vi "Steuerprogramm-11-15.vi"() -> ()   [LabVIEW 2010]
uses:
  <vilib>/rvi/interface/nirviReadWriteControl/nirviReadWriteControl.xnode
  <vilib>/rvi/errors/niLvFpgaWhatHappensToTopLevelVI.ctl
  <vilib>/rvi/interface/common/niFpgaNodeNameForErrorReporting.ctl
  <vilib>/rvi/errors/niLvFpgaAdjustHostInterfaceError.vi
  gvbooleschRT.vi
  <vilib>/functionblocks/FB Core/FB Core.xnode
  <vilib>/functionblocks/Counter/Elapsed Timer/Elapsed Timer.vi
  <vilib>/functionblocks/NI_FunctionBlock Libraries.lvlib
  <vilib>/rvi/interface/nirviCloseFPGA/nirviCloseFPGA.xnode
  <vilib>/addons/control/pid/NI_PID_pid.lvlib
  GVMWHorst.vi
  GVMethodenwechsel.vi
  GVHorstSP.vi
  GVZwangs.vi
  GVHK1Hz.vi
  GVHeizenLH.vi
  GVAIs.vi
  <vilib>/addons/control/pid/pid.llb/PID (DBL Array).vi
  GVTrapsMachs.vi
  GVaktuelleTDMS.vi
  GVECDs.vi
  GVZeitenZyklen.vi
  GVProbenvol.vi
  GVVentilposition.vi
  <vilib>/rvi/interface/nirviMethod/nirviMethod.xnode
  GVChroms.vi
  C:/Users/HAGAR-IV/Desktop/Zeugs/Johnny/pertrasgc fpga/FPGA-Programm-11-15.vi
  NiFpgaLv.dll
  <vilib>/Utility/error.llb/Error Cluster From Error Code.vi
  C:/Users/HAGAR-IV/Desktop/Zeugs/markus/version feb 2012/FPGA Bitfiles/pertrasgcfpga2_FPGATarget_FPGA-Programm-11_875D3646.lvbitx
  <vilib>/FPGAPlugInAG/cRIO-9114/niLvFpga_Close_cRIO-9114.vi
  Emil/HAGAR V - Licor/control/Licor-Sequences.ctl
  Emil/HAGAR V - Licor/control/Licor-Pump.ctl
  Emil/Licor-Steuerung/LicorLI7000/conventions/Licor-Source.ctl
  Emil/Licor-Steuerung/LicorLI7000/LicorLI7000.lvlib
panel:
  in  "Methode speichern":bool
  out "ZyklusNummernGesamt":i32[](array[numeric])
  in  "veränderte Methode benutzen":bool
  in  "Methode verändern":bool
  out "ZyklusNummern":i32[](array[numeric])
  out "Big Ben, Methodenzeit, Zykluszeit0, Zykluszeit1, Zykluszeit2A, Zykluszeit2B":i32[](array[numeric])
  in  "global stop RT":bool
  in  "Methode":i32(ring) items=["Bedingsmethode", "Startmethode", "Meßmodus", "Shut-up-Methode", "Test"]
  in  "Registerkarte":T1(tab)
  out "AIs1":dbl[](array[numeric])
  out "AIs1":string[](array[string])
  out "AIs2":string[](array[string])
  out "AIs3":string[](array[string])
  out "AIs2":dbl[](array[numeric])
  out "AIs3":dbl[](array[numeric])
  out "schnelleAnzeige":cluster{dbl[], dbl[]}(graph)
  in  "TafelWischen!":bool
  in  "dargestellte Größe 3":i32(ring)=1 items=["TemperaturTrap1[°C]", "TemperaturTrap2[°C]", "TemperaturPreMach1[°C]", "TemperaturPreMach2[°C]", "TemperaturMainMach1[°C]", "TemperaturMainMach2[°C]", "PrC0", "PrC0-Licor", "PrC1-Säule2", "PrC1-Säule1", "MFC1-Sample", "MFC1-Methan", "PrC1-BackFlush1", "PrC1-BackFlush2", "MFC2A", "MFC2B", "MFC2C", "PrC2A", "MFC2D", "MFC2E", "PrC2B"]
  in  "An/Aus":bool
  out "CO2 B 2":cluster{"t0":dbl, "dt":dbl, "Y":dbl[]}(graph)
  in  "manual control":T3={"sequence manual"=enum."WAIT", "sequence manual ?"=FALSE}
  out "raw data buffer out":string[](array[string])
  in  "command parameter":T6={"CO2 ref"=392.0, "CO2 span"=372.0, "H2O ref"=0.0, "H2O span"=0.0, "Zt"=0.0, "Zi"=1.2, "Zeitstempel"=timestamp(0 s since 1904-01-01), "Zm"=0.0, "Licor-Pump"="Off", "Licor-Sources"=["CO2A W", "CO2B W", "H2OA W", "H2OB W", "T C", "T V", "P kPa", "P V", "RH %", "CO2A um/m", "CO2B um/m", "H2OA mm/m", "H2OB mm/m"], "S"=1.0}
  out "Housekeeping1":cluster{dbl[], dbl[]}(graph)
  in  "Zeitachse1":i32(ring)=1 items=["Zykluszeit [s] Mod0", "Zykluszeit [s] Mod1", "Zykluszeit [s] Mod2A", "Zykluszeit [s] Mod2B"]
  in  "dargestellte Größe 1":i32(ring)=1 items=["T1-Trap1", "T1-Trap2", "T1-StirlingKühlkopf", "T1-PreCol1", "T1-PreCol2", "T1-MainCol1a", "T1-MainCol1b", "T1-MainCol2a", "T1-MainCol2b", "T1-Bronkhorst1a", "T1-Bronkhorst1b", "T1-Bronkhorst2a", "T1-Bronkhorst2b", "T1-2Pos1B", "T1-Spare9", "T1-2Pos1A", "T1-Spare10", "T1-TurboPump", "T1-StirlingPlatine", "T1-Spare5", "T1-Spare6", "T1-Spare7", "T1-Spare8", "F1-MFM1", "F1-MFM0D [mL]", "P1-MethaneHP", "P1-MethaneLP", "P1-Vacuum", "TurboSpeed", "I1-MS-AC", "I1-Trap1", "I1-Trap2", "T2-ECD1a", "T2-ECD1b", "T2-ECD2a", "T2-ECD2b", "T2-Col1a", "T2-Col1b", "T2-Col2a", "T2-Col2b", "T2-Spare1", "T2-Spare2", "T2-Oven_a", "T2-Oven_b", "T2-Spare3", "T2-Spare4", "T2-Spare5", "F2-MFM0", "F2-MFM2A", "F2-MFM2B", "P2-N2O_HP", "P2-N2O_LP", "P2-CO2_HP", "P2-CO2_LP", "AI-Spare1", "FL-MFM1000mL", "AI-Spare3", "AI-Spare4", "AI-Spare5", "AI-Spare6", "AI-Spare7", "AI-Spare8", "AI-Spare9", "FL-MFM30mL", "T0-DC/DC5", "I0-24V_M0", "I0-48V_M1", "I0-24V_M1", "I0-28V_M2", "T0-Spare3", "T0-Spare2", "T0-Spare4", "T0-DC/DC7", "I0-20V_Laptop", "I0-28V_M1", "I0-24V_M2", "I0-12V_Licor", "T0-Spare1", "T0-Drier", "T0-Spare5", "F0-MFM0A [L]", "TL-Licor_a", "P0-Span-HP", "P0-spare1", "P0-Stickstoff-LP", "P0-Helium-LP", "P0-Cal-HP", "P0-P9Tavco[bar]", "F0-MFM0B [L]", "TL-Licor_b", "P0-Span-LP", "P0-spare2", "P0-Stickstoff-HP", "P0-Helium-HP", "P0-Cal-LP", "F0-MFM3", "TemperaturTrap1[°C]", "TemperaturTrap2[°C]", "TemperaturPreMach1[°C]", "TemperaturPreMach2[°C]", "TemperaturMainMach1[°C]", "TemperaturMainMach2[°C]", "PrC0", "PrC0-Licor", "PrC1-Säule2", "PrC1-Säule1", "MFC1-Sample", "MFC1-Methan", "PrC1-BackFlush1", "PrC1-BackFlush2", "MFC2A", "MFC2B", "MFC2C", "PrC2A", "MFC2D", "MFC2E", "PrC2B"]
  out "Housekeeping2":cluster{dbl[], dbl[]}(graph)
  in  "Zeitachse2":i32(ring)=1 items=["Zykluszeit [s] Mod0", "Zykluszeit [s] Mod1", "Zykluszeit [s] Mod2A", "Zykluszeit [s] Mod2B"]
  in  "dargestellte Größe 2":i32(ring)=1 items=["T1-Trap1", "T1-Trap2", "T1-StirlingKühlkopf", "T1-PreCol1", "T1-PreCol2", "T1-MainCol1a", "T1-MainCol1b", "T1-MainCol2a", "T1-MainCol2b", "T1-Bronkhorst1a", "T1-Bronkhorst1b", "T1-Bronkhorst2a", "T1-Bronkhorst2b", "T1-2Pos1B", "T1-Spare9", "T1-2Pos1A", "T1-Spare10", "T1-TurboPump", "T1-StirlingPlatine", "T1-Spare5", "T1-Spare6", "T1-Spare7", "T1-Spare8", "F1-MFM1", "F1-MFM0D [mL]", "P1-MethaneHP", "P1-MethaneLP", "P1-Vacuum", "TurboSpeed", "I1-MS-AC", "I1-Trap1", "I1-Trap2", "T2-ECD1a", "T2-ECD1b", "T2-ECD2a", "T2-ECD2b", "T2-Col1a", "T2-Col1b", "T2-Col2a", "T2-Col2b", "T2-Spare1", "T2-Spare2", "T2-Oven_a", "T2-Oven_b", "T2-Spare3", "T2-Spare4", "T2-Spare5", "F2-MFM0", "F2-MFM2A", "F2-MFM2B", "P2-N2O_HP", "P2-N2O_LP", "P2-CO2_HP", "P2-CO2_LP", "AI-Spare1", "FL-MFM1000mL", "AI-Spare3", "AI-Spare4", "AI-Spare5", "AI-Spare6", "AI-Spare7", "AI-Spare8", "AI-Spare9", "FL-MFM30mL", "T0-DC/DC5", "I0-24V_M0", "I0-48V_M1", "I0-24V_M1", "I0-28V_M2", "T0-Spare3", "T0-Spare2", "T0-Spare4", "T0-DC/DC7", "I0-20V_Laptop", "I0-28V_M1", "I0-24V_M2", "I0-12V_Licor", "T0-Spare1", "T0-Drier", "T0-Spare5", "F0-MFM0A [L]", "TL-Licor_a", "P0-Span-HP", "P0-spare1", "P0-Stickstoff-LP", "P0-Helium-LP", "P0-Cal-HP", "P0-P9Tavco[bar]", "F0-MFM0B [L]", "TL-Licor_b", "P0-Span-LP", "P0-spare2", "P0-Stickstoff-HP", "P0-Helium-HP", "P0-Cal-LP", "F0-MFM3", "TemperaturTrap1[°C]", "TemperaturTrap2[°C]", "TemperaturPreMach1[°C]", "TemperaturPreMach2[°C]", "TemperaturMainMach1[°C]", "TemperaturMainMach2[°C]", "PrC0", "PrC0-Licor", "PrC1-Säule2", "PrC1-Säule1", "MFC1-Sample", "MFC1-Methan", "PrC1-BackFlush1", "PrC1-BackFlush2", "MFC2A", "MFC2B", "MFC2C", "PrC2A", "MFC2D", "MFC2E", "PrC2B"]
  out "Detektor 2":cluster{dbl[], dbl[]}[](graph)
  in  "Detektor":i32(ring) items=["ECD1", "ECD2"]
  in  "HK1YMin":dbl
  in  "HK1YMax":dbl=100.0
  in  "HK2YMin":dbl
  in  "HK2YMax":dbl=100.0
  in  "DetYMin":dbl
  in  "DetYMax":dbl=100.0
  out "Zykluslängen [s]":dbl[](array[numeric])
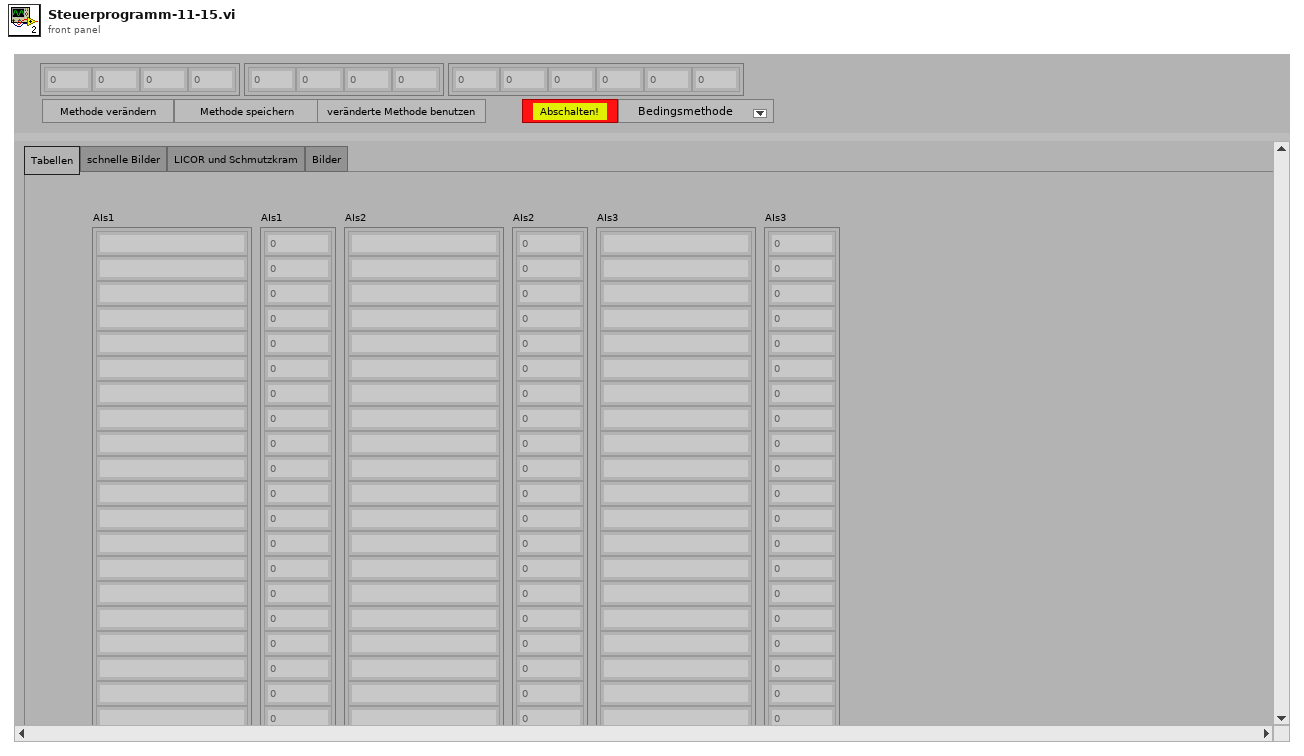
[diagram p1: front panel]
types:
  T1 = enum32{"Tabellen", "schnelle Bilder", "LICOR und Schmutzkram", "Bilder"}
  T2 = typedef "Licor-Sequences.ctl" = enum16{"test", "WAIT", "warmup", "initialize", "calibrate Z", "calibrate S"}
  T3 = cluster{"sequence manual":T2, "sequence manual ?":bool}
  T4 = typedef "Licor-Pump.ctl" = string
  T5 = typedef "LicorLI7000.lvlib/Licor-Source.ctl" = string
  T6 = cluster{"CO2 ref":dbl, "CO2 span":dbl, "H2O ref":dbl, "H2O span":dbl, "Zt":dbl, "Zi":dbl, "Zeitstempel":timestamp, "Zm":dbl, "Licor-Pump":T4, "Licor-Sources":T5[], "S":dbl}
  T7 = cluster{"Zykluslängen [s]":dbl[], "ZeitpktDIOsMod0":dbl[], "ZeitpktDIOsMod1":dbl[], "ZeitpktDIOsMod2A":dbl[], "ZeitpktDIOsMod2B":dbl[], "DIOsSPMod0":bool[][], "DIOsSPMod1":bool[][], "DIOsSPMod2A":bool[][], "DIOsSPMod2B":bool[][], "Mod0HorstZeitpkt":dbl[], "Mod1HorstZeitpkt":dbl[], "Mod2AHorstZeitpkt":dbl[], "Mod2BHorstZeitpkt":dbl[], "HorstSPMod0":dbl[][], "HorstSPMod1":dbl[][], "HorstSPMod2A":dbl[][], "HorstSPMod2B":dbl[][], "LHSetpoints":dbl[], "LHHeizen?":bool[], "ZPktFPGABoolesch":dbl[], "FPGABoolesch":bool[][], "ZeitpktFPGAPID":dbl[], "FPGAPID":cluster{"proportional gain (Kc)":fxp<+/-,16,8>, "integral gain (Kc*Ts/Ti)":fxp<+/-,16,8>, "derivative gain (Kc*Td/Ts)":fxp<+/-,16,8>}[][], "ZeitpktFPGAFixp":dbl[], "SHSetpoints":dbl[][], "t_PreMach1":dbl[], "T_PreMach1":dbl[], "t_PreMach2":dbl[], "T_PreMach2":dbl[], "PIDs für \"träge\" Heizungen":cluster{"proportional gain (Kc)":dbl, "integral time (Ti, min)":dbl, "derivative time (Td, min)":dbl}[], "Zwangsbedingungen":dbl[][], "Dateien fürs MS schicken?":bool, "ZeitpunkteMPV":dbl[], "SPMPV":i32[], "ZeitpktMS-1":dbl, "ZeitpktMS-2":dbl, "Int.Start1":dbl, "Int.Stop1":dbl, "Int.Start2":dbl, "Int.Stop2":dbl, "Methodenname":string, "t_MainMach1":dbl[], "T_MainMach1":dbl[], "t_MainMach2":dbl[], "T_MainMach2":dbl[]}[]
  T8 = cluster{"DIOsMod0Nr":i32[], "DIOsMod1Nr":i32[], "DIOsMod2ANr":i32[], "DIOsMod2BNr":i32[], "AIsLH":i32[], "Anzahl Horst/Modul":i32[], "Regler für den Probenfluß":i32, "StringSPvorgebenMod0":string[], "StringSPvorgebenMod1":string[], "StringSPvorgebenMod2A":string[], "StringSPvorgebenMod2B":string[], "StringMWAntwort0":string[], "StringMWAntwort1":string[], "StringMWAntwort2A":string[], "StringMWAntwort2B":string[], "UmrechnungHorst0":dbl[], "UmrechnungHorst1":dbl[], "UmrechnungHorst2A":dbl[], "UmrechnungHorst2B":dbl[], "StringMWabfragenMod0":string[], "StringMWabfragenMod1":string[], "StringMWabfragenMod2A":string[], "StringMWabfragenMod2B":string[], "Modul1/AI koeff":dbl[][], "Modul2/AI koeff":dbl[][], "Modul3/AI koeff":dbl[][], "Traps/MachsKoeff":dbl[][], "Modul1/AIsNamen":string[], "Modul2/AIsNamen":string[], "Modul3/AIsNamen":string[], "DIOsMod0Name":string[], "DIOsMod1Name":string[], "DIOsMod2AName":string[], "DIOsMod2BName":string[], "HorstMod0Name":string[], "HorstMod1Name":string[], "HorstMod2AName":string[], "HorstMod2BName":string[], "Startmethode":i32, "Dateiordner Housekeeping":path, "Dateiname Housekeeping":string, "DateiordnerECD1":path, "DateinameECD1":string, "DateiordnerECD2":path, "DateinameECD2":string, "NamenLangsameHeizungen":string[], "ModuleLH":i32[]}
  T9 = enum16{"open", "replace", "create", "open or create", "replace or create", "replace or create with confirmation"}
  T10 = cluster{"Zykluslängen [s]":dbl[], "ZeitpktDIOsMod0":dbl[], "ZeitpktDIOsMod1":dbl[], "ZeitpktDIOsMod2A":dbl[], "ZeitpktDIOsMod2B":dbl[], "DIOsSPMod0":bool[][], "DIOsSPMod1":bool[][], "DIOsSPMod2A":bool[][], "DIOsSPMod2B":bool[][], "Mod0HorstZeitpkt":dbl[], "Mod1HorstZeitpkt":dbl[], "Mod2AHorstZeitpkt":dbl[], "Mod2BHorstZeitpkt":dbl[], "HorstSPMod0":dbl[][], "HorstSPMod1":dbl[][], "HorstSPMod2A":dbl[][], "HorstSPMod2B":dbl[][], "LangsameHeizungenSP":dbl[], "LHHeizen?":bool[], "ZPktFPGABoolesch":dbl[], "FPGABoolesch":bool[][], "ZeitpktFPGAPID":dbl[], "FPGAPID":cluster{"proportional gain (Kc)":fxp<+/-,16,8>, "integral gain (Kc*Ts/Ti)":fxp<+/-,16,8>, "derivative gain (Kc*Td/Ts)":fxp<+/-,16,8>}[][], "ZeitpktFPGAFixp":dbl[], "FPGAFixp":fxp<+/-,16,4>[][], "ZeitpktMach1":dbl[], "TempMach1":dbl[], "ZeitpktMach2":dbl[], "TempMach2":dbl[], "PIDs für \"träge\" Heizungen":cluster{"proportional gain (Kc)":dbl, "integral time (Ti, min)":dbl, "derivative time (Td, min)":dbl}[], "Zwangsbedingungen":dbl[][], "Text0 MS-Datei":string, "Info":string, "wie wird gespeichert?":u16, "Speicherlänge":string, "Dateien fürs MS schicken?":bool, "Pfad MS-Datei CRIO":path}[]
  T11 = typedef "niFpgaNodeNameForErrorReporting.ctl" = enum16{"Open FPGA VI Reference", "Read/Write Control", "Invoke Method: Abort", "Invoke Method: Acknowledge IRQ", "Invoke Method: Download", "Invoke Method: FIFO.Configure", "Invoke Method: FIFO.Read", "Invoke Method: FIFO.Start", "Invoke Method: FIFO.Stop", "Invoke Method: FIFO.Write", "Invoke Method: Reset", "Invoke Method: Run", "Invoke Method: Wait on IRQ", "Close FPGA VI Reference"}
  T12 = typedef "niLvFpgaWhatHappensToTopLevelVI.ctl" = enum16{"top level VI scripted behind XNode", "top level VI inlined behind XNode"}
  T13 = cluster{"Zyklus1":i32, "Zeitachse1":i32, "dargestellte Größe 1":i32, "Zyklus2":i32, "Zeitachse2":i32, "dargestellte Größe 2":i32}
  T14 = cluster{"Zykluslängen [s]":dbl[], "ZeitpktDIOsMod0":dbl[], "ZeitpktDIOsMod1":dbl[], "ZeitpktDIOsMod2A":dbl[], "ZeitpktDIOsMod2B":dbl[], "DIOsSPMod0":bool[][], "DIOsSPMod1":bool[][], "DIOsSPMod2A":bool[][], "DIOsSPMod2B":bool[][], "Mod0HorstZeitpkt":dbl[], "Mod1HorstZeitpkt":dbl[], "Mod2AHorstZeitpkt":dbl[], "Mod2BHorstZeitpkt":dbl[], "HorstSPMod0":dbl[][], "HorstSPMod1":dbl[][], "HorstSPMod2A":dbl[][], "HorstSPMod2B":dbl[][], "LHSetpoints":dbl[], "LHHeizen?":bool[], "ZPktFPGABoolesch":dbl[], "FPGABoolesch":bool[][], "ZeitpktFPGAPID":dbl[], "FPGAPID":cluster{"proportional gain (Kc)":fxp<+/-,16,8>, "integral gain (Kc*Ts/Ti)":fxp<+/-,16,8>, "derivative gain (Kc*Td/Ts)":fxp<+/-,16,8>}[][], "ZeitpktFPGAFixp":dbl[], "SHSetpoints":dbl[][], "t_PreMach1":dbl[], "T_PreMach1":dbl[], "t_PreMach2":dbl[], "T_PreMach2":dbl[], "PIDs für \"träge\" Heizungen":cluster{"proportional gain (Kc)":dbl, "integral time (Ti, min)":dbl, "derivative time (Td, min)":dbl}[], "Zwangsbedingungen":dbl[][], "Dateien fürs MS schicken?":bool, "ZeitpunkteMPV":dbl[], "SPMPV":i32[], "ZeitpktMS-1":dbl, "ZeitpktMS-2":dbl, "Int.Start1":dbl, "Int.Stop1":dbl, "Int.Start2":dbl, "Int.Stop2":dbl, "Methodenname":string, "t_MainMach1":dbl[], "T_MainMach1":dbl[], "t_MainMach2":dbl[], "T_MainMach2":dbl[]}
  T15 = cluster{"DIOsMod0Name":string[], "DIOsMod1Name":string[], "DIOsMod2AName":string[], "DIOsMod2BName":string[], "HorstMod0Name":string[], "HorstMod1Name":string[], "HorstMod2AName":string[], "HorstMod2BName":string[], "NamenLangsameHeizungen":string[]}
  T16 = cluster{"Dateiordner Housekeeping":path, "DateiordnerECD1":path, "DateiordnerECD2":path, "Dateiname Housekeeping":string, "DateinameECD1":string, "DateinameECD2":string, "tdms0":refnum<k34>, "tdms1":refnum<k34>, "tdms0":refnum<k34>, "tdms1":refnum<k34>, "tdms0":refnum<k34>, "tdms1":refnum<k34>}
  T17 = cluster{"proportional gain (Kc)":fxp<+/-,16,8>, "integral gain (Kc*Ts/Ti)":fxp<+/-,16,8>, "derivative gain (Kc*Td/Ts)":fxp<+/-,16,8>}[][]
  T18 = cluster{"proportional gain (Kc)":dbl, "integral time (Ti, min)":dbl, "derivative time (Td, min)":dbl}[]
  T19 = cluster{"Heizen?LH[0]":bool, "Heizen?LH[1]":bool, "Heizen?LH[2]":bool, "Heizen?LH[3]":bool, "Heizen?LH[4]":bool, "Heizen?LH[5]":bool, "Heizen?LH[6]":bool, "Heizen?LH[7]":bool, "Heizen?LH[8]":bool, "Heizen?LH[9]":bool, "Heizen?LH[10]":bool, "Heizen?LH[11]":bool}
  T20 = cluster{"[0]":u32, "[1]":u32, "[2]":u32, "[3]":u32, "[4]":u32, "[5]":u32, "[6]":u32, "[7]":u32, "[8]":u32, "[9]":u32, "[10]":u32, "[11]":u32}
  T21 = cluster{cluster{"ZeitpktDIOsMod2B":dbl[]}[], cluster{"DIOsSPMod2B":bool[][]}[], cluster{"Mod2BHorstZeitpkt":dbl[]}[], cluster{"HorstSPMod2B":dbl[][]}[], "LHHeizen?":bool[], "ZPktFPGABoolesch":dbl[], "FPGABoolesch":bool[][], "ZeitpktFPGAPID":dbl[], "FPGAPID":cluster{"proportional gain (Kc)":fxp<+/-,16,8>, "integral gain (Kc*Ts/Ti)":fxp<+/-,16,8>, "derivative gain (Kc*Td/Ts)":fxp<+/-,16,8>}[][], "ZeitpktFPGAFixp":dbl[], "SHSetpoints":dbl[][], "t_PreMach1":dbl[], "T_PreMach1":dbl[], "t_PreMach2":dbl[], "T_PreMach2":dbl[], "ZeitpunkteMPV":dbl[], "SPMPV":i32[], "t_MainMach1":dbl[], "T_MainMach1":dbl[], "t_MainMach2":dbl[], "T_MainMach2":dbl[]}
  T22 = cluster{"Zykluslängen [s]":dbl[], "ZeitpktDIOsMod0":dbl[], "ZeitpktDIOsMod1":dbl[], "ZeitpktDIOsMod2A":dbl[], "ZeitpktDIOsMod2B":dbl[], "DIOsSPMod0":bool[][], "DIOsSPMod1":bool[][], "DIOsSPMod2A":bool[][], "DIOsSPMod2B":bool[][], "Mod0HorstZeitpkt":dbl[], "Mod1HorstZeitpkt":dbl[], "Mod2AHorstZeitpkt":dbl[], "Mod2BHorstZeitpkt":dbl[], "HorstSPMod0":dbl[][], "HorstSPMod1":dbl[][], "HorstSPMod2A":dbl[][], "HorstSPMod2B":dbl[][], "LangsameHeizungenSP":dbl[], "LHHeizen?":bool[], "ZPktFPGABoolesch":dbl[], "FPGABoolesch":bool[][], "ZeitpktFPGAPID":dbl[], "FPGAPID":cluster{"proportional gain (Kc)":fxp<+/-,16,8>, "integral gain (Kc*Ts/Ti)":fxp<+/-,16,8>, "derivative gain (Kc*Td/Ts)":fxp<+/-,16,8>}[][], "ZeitpktFPGAFixp":dbl[], "FPGAFixp":dbl[][], "t_PreMach1":dbl[], "T_PreMach1":dbl[], "t_PreMach2":dbl[], "T_PreMach2":dbl[], "PIDs für \"träge\" Heizungen":cluster{"proportional gain (Kc)":dbl, "integral time (Ti, min)":dbl, "derivative time (Td, min)":dbl}[], "Zwangsbedingungen":dbl[][], "MS-Daten?":bool, "ZeitpunkteMPV":dbl[], "SetpointMPV":i32[], "ZeitpktMS-1":dbl, "ZeitpktMS-2":dbl, "Int.Start1":dbl, "Int.Stop1":dbl, "Int.Start2":dbl, "Int.Stop2":dbl, "Methodenname":string, "t_MainMach1":dbl[], "T_MainMach1":dbl[], "t_MainMach2":dbl[], "T_MainMach2":dbl[]}
  T23 = cluster{"ZyklusNummern":i32[], "ZeilennummernDIOs":i32[], "ZwangsDIO?":cluster{bool[]}[], "ZeilennummernHorst":i32[], "ZwangsHorst?":cluster{bool[]}[], "ZeileFPGABoolesch":i32, "ZwangsFPGABoolesch?":bool[], "ZeileFPGAPID":i32, "ZeileFPGAFixp":i32, "ZeilePreMach1":i32, "ZeilePreMach2":i32, "ZeilennummerMPV":i32, "ZeileMainMach1":i32, "ZeileMainMach2":i32}
  T24 = cluster{"ZyklusNummern":i32[], i32[], "ZwangsDIO?":cluster{bool[]}[], i32[], "ZwangsHorst?":cluster{bool[]}[], i32, "ZwangsFPGABoolesch?":bool[], i32, i32, "ZeileMach":i32, "ZeileMach":i32, i32, "ZeileMach":i32, "ZeileMach":i32}
  T25 = cluster{string[], string[], string[], dbl[], dbl[], dbl[]}
  T26 = cluster{"Befehle1":string[], "Befehle2":string[], "Befehle3":string[]}
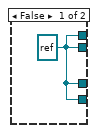
[diagram p2: hidden frame]
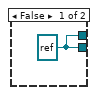
[diagram p3: hidden frame]
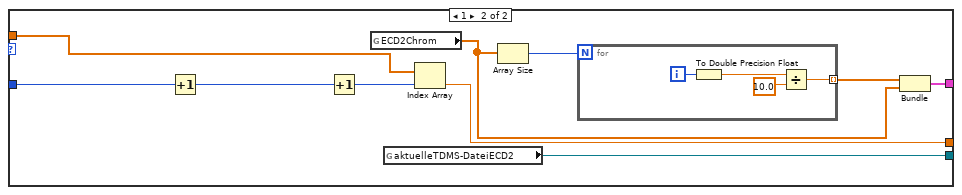
[diagram p13: hidden frame]
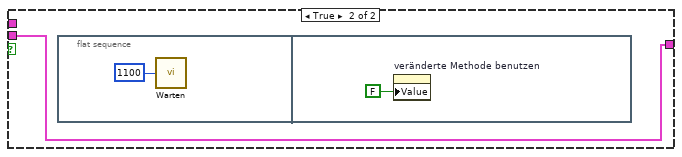
[diagram p14: hidden frame]
diagram:
  (unwired) T10 [{"Zykluslängen [s]"=[180.0, 180.0, 180.0, 180.0], "ZeitpktDIOsMod0"=[0.0, 180.0], "ZeitpktDIOsMod1"=[0.0, 2.0, 15.0, 60.0, 61.0, 70.0, 80.0, 170.0, 180.0], "ZeitpktDIOsMod2A"=[0.0, 180.0], "ZeitpktDIOsMod2B"=[0.0, 60.0, 180.0], "DIOsSPMod0"=[[FALSE], [FALSE]], "DIOsSPMod1"=[[TRUE, TRUE, FALSE, TRUE, FALSE, TRUE, TRUE, TRUE, FALSE, FALSE, TRUE, FALSE, FALSE, FALSE, FALSE, FALSE, FALSE, TRUE], [TRUE, FALSE, FALSE, TRUE, FALSE, TRUE, TRUE, TRUE, FALSE, FALSE, TRUE, FALSE, FALSE, FALSE, FALSE, FALSE, FALSE, TRUE], [TRUE, FALSE, FALSE, FALSE, FALSE, TRUE, TRUE, FALSE, FALSE, FALSE, TRUE, FALSE, FALSE, FALSE, FALSE, FALSE, TRUE, TRUE], [TRUE, FALSE, FALSE, FALSE, FALSE, FALSE, TRUE, FALSE, FALSE, FALSE, TRUE, FALSE, FALSE, FALSE, FALSE, FALSE, TRUE, TRUE], [TRUE, FALSE, FALSE, FALSE, FALSE, FALSE, TRUE, FALSE, FALSE, FALSE, TRUE, FALSE, FALSE, FALSE, FALSE, FALSE, TRUE, TRUE], [TRUE, FALSE, FALSE, FALSE, FALSE, FALSE, TRUE, FALSE, FALSE, FALSE, TRUE, FALSE, FALSE, FALSE, FALSE, FALSE, TRUE, TRUE], [TRUE, FALSE, FALSE, FALSE, FALSE, FALSE, TRUE, FALSE, FALSE, FALSE, TRUE, FALSE, FALSE, FALSE, FALSE, FALSE, FALSE, TRUE], [TRUE, FALSE, FALSE, FALSE, FALSE, FALSE, TRUE, FALSE, FALSE, FALSE, TRUE, FALSE, FALSE, FALSE, FALSE, FALSE, FALSE, TRUE], [TRUE, FALSE, FALSE, FALSE, FALSE, FALSE, TRUE, FALSE, FALSE, FALSE, TRUE, FALSE, FALSE, FALSE, FALSE, FALSE, FALSE, TRUE]], "DIOsSPMod2A"=[[FALSE], [FALSE]], "DIOsSPMod2B"=[[FALSE], [FALSE]], "Mod0HorstZeitpkt"=[0.0, 180.0], "Mod1HorstZeitpkt"=[0.0, 55.0, 75.0, 180.0], "Mod2AHorstZeitpkt"=[0.0, 20.0, 180.0], "Mod2BHorstZeitpkt"=[0.0, 380.0], "HorstSPMod0"=[[2.66], [2.66]], "HorstSPMod1"=[[1.9, 0.0, 1.2], [0.0, 0.0, 1.2], [1.9, 0.0, 1.2], [1.9, 0.0, 1.2]], "HorstSPMod2A"=[[300.0], [300.0], [300.0]], "HorstSPMod2B"=[[0.0], [0.0]], "LangsameHeizungenSP"=[60.0, 220.0, 120.0, 60.0, 110.0, 0.0], "LHHeizen?"=[FALSE, TRUE, TRUE, FALSE, TRUE, FALSE], "ZPktFPGABoolesch"=[0.0, 60.0, 75.0, 180.0], "FPGABoolesch"=[[FALSE, FALSE, FALSE, FALSE, TRUE, FALSE], [FALSE, FALSE, TRUE, FALSE, TRUE, FALSE], [FALSE, FALSE, FALSE, FALSE, TRUE, FALSE], [FALSE, FALSE, FALSE, FALSE, TRUE, FALSE]], "ZeitpktFPGAPID"=[0.0, 60.0, 180.0], "FPGAPID"=[[{"proportional gain (Kc)"=5.0, "integral gain (Kc*Ts/Ti)"=0.0, "derivative gain (Kc*Td/Ts)"=0.0}, {"proportional gain (Kc)"=1.0, "integral gain (Kc*Ts/Ti)"=1.66796875, "derivative gain (Kc*Td/Ts)"=0.0}, {"proportional gain (Kc)"=5.0, "integral gain (Kc*Ts/Ti)"=0.03515625, "derivative gain (Kc*Td/Ts)"=0.0234375}, {"proportional gain (Kc)"=1.0, "integral gain (Kc*Ts/Ti)"=1.66796875, "derivative gain (Kc*Td/Ts)"=0.0}], [{"proportional gain (Kc)"=5.0, "integral gain (Kc*Ts/Ti)"=0.0, "derivative gain (Kc*Td/Ts)"=0.0}, {"proportional gain (Kc)"=1.0, "integral gain (Kc*Ts/Ti)"=1.66796875, "derivative gain (Kc*Td/Ts)"=0.0}, {"proportional gain (Kc)"=5.0, "integral gain (Kc*Ts/Ti)"=0.03515625, "derivative gain (Kc*Td/Ts)"=0.0234375}, {"proportional gain (Kc)"=1.0, "integral gain (Kc*Ts/Ti)"=1.66796875, "derivative gain (Kc*Td/Ts)"=0.0}], [{"proportional gain (Kc)"=0.0, "integral gain (Kc*Ts/Ti)"=0.0, "derivative gain (Kc*Td/Ts)"=0.0}, {"proportional gain (Kc)"=0.0, "integral gain (Kc*Ts/Ti)"=0.0, "derivative gain (Kc*Td/Ts)"=0.0}, {"proportional gain (Kc)"=2.0, "integral gain (Kc*Ts/Ti)"=0.03125, "derivative gain (Kc*Td/Ts)"=0.01953125}, {"proportional gain (Kc)"=0.0, "integral gain (Kc*Ts/Ti)"=0.0, "derivative gain (Kc*Td/Ts)"=0.0}], [{"proportional gain (Kc)"=0.0, "integral gain (Kc*Ts/Ti)"=0.0, "derivative gain (Kc*Td/Ts)"=0.0}, {"proportional gain (Kc)"=0.0, "integral gain (Kc*Ts/Ti)"=0.0, "derivative gain (Kc*Td/Ts)"=0.0}, {"proportional gain (Kc)"=2.0, "integral gain (Kc*Ts/Ti)"=0.03125, "derivative gain (Kc*Td/Ts)"=0.01953125}, {"proportional gain (Kc)"=0.0, "integral gain (Kc*Ts/Ti)"=0.0, "derivative gain (Kc*Td/Ts)"=0.0}], [{"proportional gain (Kc)"=0.0, "integral gain (Kc*Ts/Ti)"=0.0, "derivative gain (Kc*Td/Ts)"=0.0}, {"proportional gain (Kc)"=0.0, "integral gain (Kc*Ts/Ti)"=0.0, "derivative gain (Kc*Td/Ts)"=0.0}, {"proportional gain (Kc)"=2.0, "integral gain (Kc*Ts/Ti)"=0.03125, "derivative gain (Kc*Td/Ts)"=0.01953125}, {"proportional gain (Kc)"=0.0, "integral gain (Kc*Ts/Ti)"=0.0, "derivative gain (Kc*Td/Ts)"=0.0}]], "ZeitpktFPGAFixp"=[0.0, 60.0, 75.0, 180.0], "FPGAFixp"=[[0.0, 0.0, 0.0, 0.0, 0.0, 0.0, 2.85009765625, 0.0], [4.59423828125, 4.599365234375, 1.699951171875, 0.0, 0.0, 0.0, 2.85009765625, 0.0], [0.0, 0.0, 0.0, 0.0, 0.0, 0.0, 2.85009765625, 0.0], [0.0, 0.0, 0.0, 0.0, 0.0, 0.0, 2.85009765625, 0.0]], "ZeitpktMach1"=[0.0, 1.0, 100.0, 101.0, 177.0, 178.0, 180.0], "TempMach1"=[50.0, 50.0, 50.0, 250.0, 250.0, 50.0, 50.0], "ZeitpktMach2"=[0.0, 0.0, 120.0], "TempMach2"=[0.0, 0.0, 0.0], "PIDs für \"träge\" Heizungen"=[{"proportional gain (Kc)"=1.0, "integral time (Ti, min)"=0.01, "derivative time (Td, min)"=0.0}, {"proportional gain (Kc)"=2.0, "integral time (Ti, min)"=1.0, "derivative time (Td, min)"=0.0}, {"proportional gain (Kc)"=4.0, "integral time (Ti, min)"=1.0, "derivative time (Td, min)"=0.0}, {"proportional gain (Kc)"=1.0, "integral time (Ti, min)"=0.01, "derivative time (Td, min)"=0.0}, {"proportional gain (Kc)"=2.0, "integral time (Ti, min)"=0.0, "derivative time (Td, min)"=0.0}, {"proportional gain (Kc)"=1.0, "integral time (Ti, min)"=0.01, "derivative time (Td, min)"=0.0}], "Zwangsbedingungen"=[[3.0, 4.0, 100.0, 23.0, 4.0, 200.0, 0.0, 0.0]], "Text0 MS-Datei"="text0", "Info"="info", "wie wird gespeichert?"=0, "Speicherlänge"="100", "Dateien fürs MS schicken?"=FALSE, "Pfad MS-Datei CRIO"=path "c:/"}] ("Eingang 2")
  n1 = Open/Create/Replace File(file path (use dialog)=path "c:/einstellungen.per" ("Datei (Dialog verwenden)"), operation (0:open)=T9."open" ("Operation (0:Öffnen)")) -> (refnum out=w11:refnum<file>)  [unwired: 4 in, 2 out]
  n2 = Open/Create/Replace File(file path (use dialog)=path "c:/methoden.per" ("Datei (Dialog verwenden)"), operation (0:open)=T9."open" ("Operation (0:Öffnen)")) -> (refnum out=w6:refnum<file>)  [unwired: 4 in, 2 out]
  n3 = Read from Binary File(5:T8 {"DIOsMod0Nr"=[], "DIOsMod1Nr"=[], "DIOsMod2ANr"=[], "DIOsMod2BNr"=[], "AIsLH"=[], "Anzahl Horst/Modul"=[], "Regler für den Probenfluß"=0, "StringSPvorgebenMod0"=[], "StringSPvorgebenMod1"=[], "StringSPvorgebenMod2A"=[], "StringSPvorgebenMod2B"=[], "StringMWAntwort0"=[], "StringMWAntwort1"=[], "StringMWAntwort2A"=[], "StringMWAntwort2B"=[], "UmrechnungHorst0"=[], "UmrechnungHorst1"=[], "UmrechnungHorst2A"=[], "UmrechnungHorst2B"=[], "StringMWabfragenMod0"=[], "StringMWabfragenMod1"=[], "StringMWabfragenMod2A"=[], "StringMWabfragenMod2B"=[], "Modul1/AI koeff"=[], "Modul2/AI koeff"=[], "Modul3/AI koeff"=[], "Traps/MachsKoeff"=[], "Modul1/AIsNamen"=[], "Modul2/AIsNamen"=[], "Modul3/AIsNamen"=[], "DIOsMod0Name"=[], "DIOsMod1Name"=[], "DIOsMod2AName"=[], "DIOsMod2BName"=[], "HorstMod0Name"=[], "HorstMod1Name"=[], "HorstMod2AName"=[], "HorstMod2BName"=[], "Startmethode"=0, "Dateiordner Housekeeping"=path "", "Dateiname Housekeeping"="", "DateiordnerECD1"=path "", "DateinameECD1"="", "DateiordnerECD2"=path "", "DateinameECD2"="", "NamenLangsameHeizungen"=[], "ModuleLH"=[]} ("Einstellungen"), 11:w11) -> (2:w9:T8, 3:w10:refnum<file>)  [unwired: 4 in, 2 out]
  n4 = Read from Binary File(5:T7 [], 11:w6) -> (2:w3:T7, 3:w5:refnum<file>)  [unwired: 4 in, 2 out]
  n5 = Close File(refnum=w10) -> ()  [unwired: 1 in, 2 out]
  n6 = Close File(refnum=w5) -> ()  [unwired: 1 in, 2 out]
  n7 = flat-sequence {
    tunnel: [w41] -> w39
    tunnel: [w47] -> w38
    tunnel: [w196] -> w36
    tunnel: [w193] -> w35
    tunnel: [w195] -> w34
    tunnel: [w187] -> w33
    tunnel: [w194] -> w32
    tunnel: [w106] -> w31
    tunnel: [w186] -> w30
    tunnel: [w185] -> w29
    tunnel: [w179] -> w28
    tunnel: [w109] -> w27
    tunnel: [w82] -> w26
    tunnel: [w192] -> w25
    tunnel: [w184] -> w24
    tunnel: [w183] -> w23
    tunnel: [w175] -> w22
    tunnel: [w174] -> w21
    tunnel: [w173] -> w20
    tunnel: [w172] -> w19
    tunnel: [w171] -> w18
    tunnel: [w170] -> w17
    tunnel: [w167] -> w16
    tunnel: [w149] -> w15
    tunnel: w9 -> [w105]
    tunnel: [w148] -> w14
    tunnel: w3 -> [w48]
    tunnel: [w47] -> w2
    tunnel: w39 -> [w260]
    tunnel: w38 -> [w333]
    tunnel: [w260] -> w37
    tunnel: w36 -> [_]
    tunnel: w35 -> [w291]
    tunnel: w34 -> [w290]
    tunnel: w33 -> [w292]
    tunnel: w32 -> [w289]
    tunnel: w31 -> [w264]
    tunnel: w30 -> [w259]
    tunnel: w29 -> [w254]
    tunnel: w28 -> [w251]
    tunnel: w27 -> [w252]
    tunnel: w26 -> [w255]
    tunnel: w25 -> [w331]
    tunnel: w24 -> [w262]
    tunnel: w23 -> [w332]
    tunnel: w22 -> [w233]
    tunnel: w21 -> [w232]
    tunnel: w20 -> [w231]
    tunnel: w19 -> [w329]
    tunnel: w18 -> [w328]
    tunnel: w17 -> [w327]
    tunnel: w16 -> [w281]
    tunnel: w15 -> [w263]
    tunnel: w14 -> [w250]
    tunnel: w3 -> [w249]
    tunnel: w2 -> [w247]
    tunnel: w37 -> [w1203]
    frame #0 {
      w49 = TRUE
      w64 = 0.0 ("Probenvol.1")
      w71 = dbl[] [-1.0] ("ECD1MW")
      w72 = FALSE ("ECD1Empfangen?")
      w63 = string[] ["TemperaturTrap1[°C]", "TemperaturTrap2[°C]", "TemperaturPreMach1[°C]", "TemperaturPreMach2[°C]", "TemperaturMainMach1[°C]", "TemperaturMainMach2[°C]"]
      w190 = string[] ["Big Ben [s]", "Methodenzeit [s]", "Zykluszeit [s] Mod0", "Zykluszeit [s] Mod1", "Zykluszeit [s] Mod2A", "Zykluszeit [s] Mod2B"]
      w180 = FALSE ("Undefinierte Werte möglich")
      w181 = FALSE ("global stop RT")
      n8 = for {
        tunnel: [w224] -> w188 mode=indexing
        tunnel: w48 -> [w225] mode=indexing
        n9 = Unbundle(w225) -> ("Methodenname"=w224:string)  [unwired: 44 out]
      }
      n10 = Unbundle(w105) -> ("DIOsMod0Nr"=w92:i32[], "DIOsMod1Nr"=w91:i32[], "DIOsMod2ANr"=w90:i32[], "DIOsMod2BNr"=w89:i32[], "AIsLH"=w79:i32[], "Anzahl Horst/Modul"=w82:i32[], "Regler für den Probenfluß"=w148:i32, "StringSPvorgebenMod0"=w147:string[], "StringSPvorgebenMod1"=w146:string[], "StringSPvorgebenMod2A"=w145:string[], "StringSPvorgebenMod2B"=w144:string[], "StringMWAntwort0"=w143:string[], "StringMWAntwort1"=w142:string[], "StringMWAntwort2A"=w141:string[], "StringMWAntwort2B"=w140:string[], "UmrechnungHorst0"=w139:dbl[], "UmrechnungHorst1"=w138:dbl[], "UmrechnungHorst2A"=w137:dbl[], "UmrechnungHorst2B"=w136:dbl[], "StringMWabfragenMod0"=w135:string[], "StringMWabfragenMod1"=w134:string[], "StringMWabfragenMod2A"=w133:string[], "StringMWabfragenMod2B"=w132:string[], "Modul1/AI koeff"=w131:dbl[][], "Modul2/AI koeff"=w130:dbl[][], "Modul3/AI koeff"=w129:dbl[][], "Traps/MachsKoeff"=w128:dbl[][], "Modul1/AIsNamen"=w127:string[], "Modul2/AIsNamen"=w126:string[], "Modul3/AIsNamen"=w125:string[], "DIOsMod0Name"=w124:string[], "DIOsMod1Name"=w123:string[], "DIOsMod2AName"=w122:string[], "DIOsMod2BName"=w121:string[], "HorstMod0Name"=w120:string[], "HorstMod1Name"=w119:string[], "HorstMod2AName"=w118:string[], "HorstMod2BName"=w117:string[], "Startmethode"=w47:i32, "Dateiordner Housekeeping"=w116:path, "Dateiname Housekeeping"=w115:string, "DateiordnerECD1"=w114:path, "DateinameECD1"=w113:string, "DateiordnerECD2"=w112:path, "DateinameECD2"=w111:string, "NamenLangsameHeizungen"=w110:string[], "ModuleLH"=w104:i32[])
      n11 = Initialize Array(0, 4 ("Dimension")) -> (w65:i32[])
      n12 = Initialize Array(0.0 ("Element"), 6 ("Dimension")) -> (w68:dbl[])
      n13 = global write "GVMethodenwechsel.vi" "Methodenwechsel?"(FALSE ("Methodenwechsel?")) -> ()
      n14 = Index Array(array=w48, index=w47) -> (element=w46:T14)
      n15 = Unbundle(w46) -> ("SPMPV"=w45:i32[])  [unwired: 44 out]
      n16 = Index Array(array=w45, index=0) -> (element=w43:i32)
      n17 = global write "GVVentilposition.vi" "Ventilposition"(w43) -> ()
      n18 = global write "GVProbenvol.vi" "Probenvol.1"(w64) -> ()
      n19 = global write "GVProbenvol.vi" "Probenvol.2"(w64) -> ()
      n20 = global write "GVECDs.vi" "ECD1MW"(w71) -> ()
      n21 = global write "GVECDs.vi" "ECD2MW"(w71) -> ()
      n22 = global write "GVECDs.vi" "ECD1Empfangen?"(w72) -> ()
      n23 = global write "GVECDs.vi" "ECD2Empfangen?"(w72) -> ()
      n24 = property on="dargestellte Größe 2" class="Ring (strict)"("AllowUndefVals"=w180) -> ()  [unwired: 2 in, 2 out]
      n25 = property on="Zeitachse2" class="Ring (strict)"("AllowUndefVals"=w180) -> ()  [unwired: 2 in, 2 out]
      n26 = property on="Zeitachse1" class="Ring (strict)"("AllowUndefVals"=w180) -> ()  [unwired: 2 in, 2 out]
      n27 = property on="dargestellte Größe 1" class="Ring (strict)"("AllowUndefVals"=w180) -> ()  [unwired: 2 in, 2 out]
      n28 = property on="Methode" class="Ring (strict)"("AllowUndefVals"=w180) -> ()  [unwired: 2 in, 2 out]
      n29 = local write "global stop RT"(w181) -> ()
      n30 = global write "gvbooleschRT.vi" "global stop RT"(w181) -> ()
      n31 = global write "GVZeitenZyklen.vi" "ZyklusNummern"(w65) -> ()
      n32 = global write "GVZeitenZyklen.vi" "ZyklusNummernGesamt"(w65) -> ()
      n33 = global write "GVZeitenZyklen.vi" "Big Ben, Methodenzeit, Zykluszeit0, Zykluszeit1, Zykluszeit2A, Zykluszeit2B"(w68) -> ()
      n34 = property on="Methode" class="Ring (strict)"("Value"=w47) -> ()  [unwired: 2 in, 2 out]
      n35 = Initialize Array(-1.0 ("Element"), 6 ("Dimension")) -> (w75:dbl[])
      n36 = Initialize Array(FALSE, 10 ("Dimension")) -> (w83:bool[])
      n37 = Initialize Array(-1.0 ("Element"), 96 ("Dimension")) -> (w76:dbl[])
      n38 = global write "GVZwangs.vi" "ZwangsFPGABoolesch!"(w83) -> ()
      n39 = global write "GVZwangs.vi" "ZwangsFPGABoolesch?"(w83) -> ()
      n40 = global write "GVTrapsMachs.vi" "Traps/Machs"(w75) -> ()
      n41 = global write "GVAIs.vi" "AIs"(w76) -> ()
      n42 = case shown="True" w49 {
        tunnel: [w218 w223] -> w166
        tunnel: [w218 w222] -> w165
        tunnel: w116 -> [_ w221]
        tunnel: w115 -> [_ w220]
        tunnel: w47 -> [_ w219]
        frame False {
          w218 = refnum<k34> refnum ("tdms1")
        }
        frame True {
          n43 = call "TDMS0.vi"("Startmethode"=w219, "Dateiname"=w220, "Dateiordner"=w221) -> ("tdms1"=w222:refnum<k34>, "tdms0"=w223:refnum<k34>)
          n44 = global write "GVaktuelleTDMS.vi" "aktuelleTDMS-DateiHK"(w223) -> ()
        }
      }
      n45 = case shown="True" w49 {
        tunnel: [w208 w217] -> w164
        tunnel: [w208 w216] -> w163
        tunnel: [w208 w215] -> w162
        tunnel: [w208 w214] -> w161
        tunnel: w114 -> [_ w213]
        tunnel: w113 -> [_ w212]
        tunnel: w112 -> [_ w211]
        tunnel: w111 -> [_ w210]
        tunnel: w47 -> [_ w209]
        frame False {
          w208 = refnum<k34> refnum ("tdms0")
        }
        frame True {
          n46 = call "TDMS0.vi"("Startmethode"=w209, "Dateiname"=w212, "Dateiordner"=w213) -> ("tdms1"=w216:refnum<k34>, "tdms0"=w217:refnum<k34>)
          n47 = call "TDMS0.vi"("Startmethode"=w209, "Dateiname"=w210, "Dateiordner"=w211) -> ("tdms1"=w214:refnum<k34>, "tdms0"=w215:refnum<k34>)
          n48 = global write "GVaktuelleTDMS.vi" "aktuelleTDMS-DateiECD1"(w217) -> ()
          n49 = global write "GVaktuelleTDMS.vi" "aktuelleTDMS-DateiECD2"(w215) -> ()
        }
      }
      n50 = for {
        tunnel: w82 -> [w202] mode=indexing
        tunnel: [w199] -> w81 mode=indexing
        tunnel: [w197] -> w80 mode=indexing
        n51 = Initialize Array(0.0 ("Element"), w202) -> (w200:dbl[])
        n52 = Initialize Array(FALSE, w202) -> (w198:bool[])
        n53 = Bundle(w200) -> (w199:cluster{dbl[]})  [unwired: 1 in]
        n54 = Bundle(w198) -> (w197:cluster{bool[]})  [unwired: 1 in]
      }
      n55 = Bundle("DIOsMod0Name"=w124, "DIOsMod1Name"=w123, "DIOsMod2AName"=w122, "DIOsMod2BName"=w121, "HorstMod0Name"=w120, "HorstMod1Name"=w119, "HorstMod2AName"=w118, "HorstMod2BName"=w117, "NamenLangsameHeizungen"=w110) -> (w183:T15)  [unwired: 1 in]
      n56 = Build Array (concatenate)(w120, w119, w118, w117) -> (w62:string[])
      n57 = Build Array (concatenate)(w147, w146, w145, w144) -> (w195:string[])
      n58 = Build Array (concatenate)(w139, w138, w137, w136) -> (w187:dbl[])
      n59 = Build Array (concatenate)(w135, w134, w133, w132) -> (w193:string[])
      n60 = Build Array (concatenate)(w143, w142, w141, w140) -> (w194:string[])
      n61 = Build Array(w92, w91, w90, w89) -> (w88:i32[][])
      n62 = Array Size(array=w110) -> (size(s)=w109:i32)
      n63 = Add Array Elements(numeric array=w82) -> (sum=w179:i32)
      n64 = Array Size(array=w79) -> (size(s)=w78:i32)
      n65 = Add Array Elements(numeric array=w82) -> (sum=w94:i32)
      n66 = Build Cluster Array(w92, w91, w90, w89) -> (w186:cluster{"DIOsMod2BNr":i32[]}[])
      n67 = Decrement(x=w104) -> (x-1=w103:i32[])
      n68 = Build Array (concatenate)(w127, w126, w125) -> (w53:string[])
      n69 = Index Array(array=w128, index (col)=0 ("Deaktivierter Index (Spalte)")) -> (element=w173:dbl[])  [unwired: 1 in]
      n70 = Index Array(array=w128, index (col)=1 ("Deaktivierter Index (Spalte)")) -> (element=w174:dbl[])  [unwired: 1 in]
      n71 = Index Array(array=w128, index (col)=2 ("Deaktivierter Index (Spalte)")) -> (element=w175:dbl[])  [unwired: 1 in]
      n72 = for {
        tunnel: w186 -> [w227] mode=indexing
        tunnel: [w228] -> w185 mode=indexing
        n73 = Unbundle(w227) -> ("DIOsMod2BNr"=w226:i32[])
        n74 = Array Size(array=w226) -> (size(s)=w228:i32)
      }
      n75 = property on="Methode" class="Ring (strict)"("Strings []"=w188) -> ()  [unwired: 2 in, 2 out]
      n76 = Build Array (concatenate)(w76, w75) -> (w74:dbl[])
      n77 = Array Size(array=w88) -> (size(s)=w87:i32[])
      n78 = Open/Create/Replace File(file path (use dialog)=path "c:/fromcriordy.txt" ("Dateipfad (Dialog verwenden)"), operation (0:open)=T9."replace or create" ("Operation (0:Öffnen)")) -> (refnum out=w152:refnum<file>, error out=w153:errorcluster)  [unwired: 4 in, 1 out]
      n79 = Initialize Array(0.0 ("Element"), w94) -> (w93:dbl[])
      n80 = Initialize Array(FALSE, w78) -> (w73:bool[])
      n81 = Multiply(x=w103, y=32) -> (x*y=w107:i32[])
      n82 = Initialize Array(-1.0, w94) -> (w96:dbl[])
      n83 = Array Subset(array=w53, index=0 ("Index"), length=32 ("Länge")) -> (→"AIs1":string[])
      n84 = Array Subset(array=w53, index=64 ("Index"), length=32 ("Länge")) -> (→"AIs3":string[])
      n85 = Array Subset(array=w53, index=32 ("Index"), length=32 ("Länge")) -> (→"AIs2":string[])
      n86 = global write "GVHK1Hz.vi" "Mod1Mod2Mod3/AITrapsMachs1Hz"(w74) -> ()
      n87 = global write "GVHeizenLH.vi" "Heizen?LH"(w73) -> ()
      n88 = global write "GVZwangs.vi" "ZwangsLangsameH!"(w73) -> ()
      n89 = global write "GVHorstSP.vi" "HorstSP"(w93) -> ()
      n90 = for {
        tunnel: w87 -> [w207] mode=indexing
        tunnel: [w204] -> w86 mode=indexing
        n91 = Initialize Array(FALSE, w207) -> (w205:bool[])
        n92 = Bundle(w205) -> (w204:cluster{bool[]})  [unwired: 1 in]
      }
      n93 = global write "GVZwangs.vi" "ZwangsLangsameH?"(w73) -> ()
      n94 = Add(x=w107, y=w79) -> (x+y=w106:i32[])
      n95 = Close File(refnum=w152, error in=w153) -> (path=w184:path)  [unwired: 1 out]
      n96 = global write "GVMWHorst.vi" "MWHorst"(w96) -> ()
      n97 = Build Array (concatenate)(string[] ["Datei Nr.", "Zyklusnr. Mod0", "Zyklusnr. Mod1", "Zyklusnr. Mod2A", "Zyklusnr. Mod2B"], w190, w53, w63, w62, "Probenvolumen1", "Probenvolumen2") -> (w192:string[])
      n98 = Build Array (concatenate)(w63, w62) -> (w61:string[])
      n99 = Build Array (concatenate)(w53, w63, w62) -> (w60:string[])
      n100 = Split 1D Array(array=w190, index=2 ("Index")) -> (second subarray=w182:string[])  [unwired: 1 out]
      n101 = property on="Zeitachse2" class="Ring (strict)"("Strings []"=w182) -> ()  [unwired: 2 in, 2 out]
      n102 = property on="Zeitachse1" class="Ring (strict)"("Strings []"=w182) -> ()  [unwired: 2 in, 2 out]
      n103 = property on="dargestellte Größe 3" class="Ring (strict)"("Strings []"=w61) -> ()  [unwired: 2 in, 2 out]
      n104 = property on="dargestellte Größe 1" class="Ring (strict)"("Strings []"=w60) -> ()  [unwired: 2 in, 2 out]
      n105 = global write "GVZwangs.vi" "ZwangsHorst!"(w81) -> ()
      n106 = global write "GVZwangs.vi" "ZwangsHorst?"(w80) -> ()
      n107 = property on="dargestellte Größe 2" class="Ring (strict)"("Strings []"=w60) -> ()  [unwired: 2 in, 2 out]
      n108 = global write "GVZwangs.vi" "ZwangsDIO!"(w86) -> ()
      n109 = global write "GVZwangs.vi" "ZwangsDIO?"(w86) -> ()
      n110 = Bundle("Dateiordner Housekeeping"=w116, "DateiordnerECD1"=w114, "DateiordnerECD2"=w112, "Dateiname Housekeeping"=w115, "DateinameECD1"=w113, "DateinameECD2"=w111, "tdms0"=w166, "tdms1"=w165, "tdms0"=w164, "tdms1"=w163, "tdms0"=w162, "tdms1"=w161) -> (w167:T16)  [unwired: 1 in]
      n111 = call "FPGA-Start-11-15.vi"() -> ("error out"=w196:errorcluster, "FPGA VI Reference Out"=w42:refnum<k20>)  [unwired: 2 in]
      n112 = Open/Create/Replace File(file path (use dialog)=path "c:/fromcriocmd.txt" ("Pfad MS-Datei CRIO"), operation (0:open)=T9."replace or create" ("Operation (0:Öffnen)")) -> (refnum out=w158:refnum<file>, error out=w157:errorcluster)  [unwired: 4 in, 1 out]
      n113 = Write to Text File(file (use dialog)=w158, text="time=yyyymmddhhmmss\ncycle=005\ninfo=1234567890123456789012345678901234567890123456789012345678901234567890123456789012345678901234567890\nlength=100\ncmd=cycle" ("Text0 MS-Datei"), error in=w157) -> (refnum out=w155:refnum<file>, error out=w154:errorcluster)  [unwired: 1 in, 1 out]
      n114 = call "MPVSenden-11-15.vi"("Ventilposition"=0, "FPGA VI Reference In"=w42) -> ("FPGA VI Reference Out"=w41:refnum<k20>)  [unwired: 1 out]
      n115 = call "AIKoeffSortieren.vi"("Modul3/AI koeff"=w129, "Modul2/AI koeff"=w130, "Modul1/AI koeff"=w131) -> ("P0"=w170:dbl[], "P1"=w171:dbl[], "P2"=w172:dbl[])
      n116 = Close File(refnum=w155, error in=w154) -> (path=w149:path)  [unwired: 1 out]
    }
    frame #1 {
      w234 = dbl[] [-1.0]
      w307 = 0
      w282 = 0 ("Zyklusnummer1")
      n117 = while {
        stop <- w1184 stop-if-true
        w1178 = 10.0
        n118 = call "Warten2"("Count(mSec)"=u32 1000) -> ()  [unwired: 1 out]
        n119 = global read "gvbooleschRT.vi" "global stop RT"() -> (w1184:bool)
        n120 = global read "GVTrapsMachs.vi" "Traps/Machs"() -> (w1174:dbl[])
        n121 = global read "GVAIs.vi" "AIs"() -> (w1175:dbl[])
        n122 = for {
          N: 9 -> [_]
          shift-right: [w1187] -> w1181
          shift-left: w1175 -> [w1188]
          shift-right: [w1185] -> w1179
          shift-left: w1174 -> [w1186]
          n123 = flat-sequence {
            tunnel: w1188 -> [w1195]
            tunnel: [w1194] -> w1187
            tunnel: w1186 -> [w1193]
            tunnel: [w1192] -> w1185
            frame #0 {
              n124 = call "Warten28"("Count(mSec)"=u32 100) -> ()  [unwired: 1 out]
            }
            frame #1 {
              n125 = global read "GVAIs.vi" "AIs"() -> (w1191:dbl[])
              n126 = Add(x=w1195, y=w1191) -> (x+y=w1194:dbl[])
              n127 = global read "GVTrapsMachs.vi" "Traps/Machs"() -> (w1190:dbl[])
              n128 = Add(x=w1190, y=w1193) -> (x+y=w1192:dbl[])
            }
          }
        }
        n129 = Divide(x=w1181, y=w1178) -> (x/y=w1180:dbl[])
        n130 = Divide(x=w1179, y=w1178) -> (x/y=w1177:dbl[])
        n131 = Build Array (concatenate)(w1180, w1177) -> (w1176:dbl[])
        n132 = global write "GVHK1Hz.vi" "Mod1Mod2Mod3/AITrapsMachs1Hz"(w1176) -> ()
      }
      n133 = while {
        tunnel: w260 -> [w665]
        tunnel: w329 -> [w664]
        tunnel: w328 -> [w663]
        tunnel: w327 -> [w662]
        stop <- w666 stop-if-true
        n134 = call "AIsFIFORT-11-15.vi"("P0"=w662, "P1"=w663, "P2"=w664, "FPGA VI Reference In"=w665) -> ()  [unwired: 1 in]
        n135 = global read "gvbooleschRT.vi" "global stop RT"() -> (w666:bool)
      }
      n136 = while {
        tunnel: w260 -> [w668]
        tunnel: w233 -> [w667]
        tunnel: w232 -> [w670]
        tunnel: w231 -> [w669]
        stop <- w672 stop-if-true
        n137 = call "TrapsMachMitteln-11-15.vi"("Traps/MachKoeff0"=w669, "Traps/MachKoeff1"=w670, "Traps/MachKoeff2"=w667, "FPGA VI Reference In"=w668) -> ()  [unwired: 1 in]
        n138 = call "Bis zum nächsten Vielfachen warten16"("Count(mSec)"=u32 100) -> ()  [unwired: 1 out]
        n139 = global read "gvbooleschRT.vi" "global stop RT"() -> (w672:bool)
      }
      n140 = while {
        shift-right: ["Methode"] -> _
        shift-left: w333 -> [w1198]
        stop <- w1200 stop-if-true
        n141 = call "Bis zum nächsten Vielfachen warten7"("Count(mSec)"=u32 1000) -> ()  [unwired: 1 out]
        n142 = global read "gvbooleschRT.vi" "global stop RT"() -> (w1200:bool)
        n143 = Not Equal?(x=w1198, y="Methode") -> (x != y?=w1196:bool)
        n144 = global write "GVMethodenwechsel.vi" "Methodenwechsel?"(w1196) -> ()
      }
      n145 = Add Array Elements(numeric array=w254) -> (sum=w253:i32)
      n146 = Array Size(array=w264) -> (size(s)=w285:i32)
      n147 = Unbundle(w281) -> ("Dateiordner Housekeeping"=w280:path, "DateiordnerECD1"=w278:path, "DateiordnerECD2"=w277:path, "Dateiname Housekeeping"=w279:string, "DateinameECD1"=w276:string, "DateinameECD2"=w275:string, "tdms0"=w274:refnum<k34>, "tdms1"=w273:refnum<k34>, "tdms0"=w272:refnum<k34>, "tdms1"=w271:refnum<k34>, "tdms0"=w270:refnum<k34>, "tdms1"=w269:refnum<k34>)
      n148 = Index Array(array=w255, index #1=0 ("Index"), index #2=1 ("Index"), index #3=2 ("Index"), index #4=3 ("Index")) -> (element #1=w296:i32, element #2=w295:i32, element #3=w298:i32, element #4=w297:i32)
      n149 = call <vilib>:"Space Constant.vi"() -> ("String"=w240:string)
      n150 = case shown="True" TRUE ("ECDSpeichern") {
        frame False {
        }
        frame True {
          w603 = dbl[] []
          n151 = global read "GVaktuelleTDMS.vi" "aktuelleTDMS-DateiECD1"() -> (w604:refnum<k34>)
          n152 = while {
            shift-right: [w612] -> _
            shift-left: w603 -> [w616]
            shift-right: [w605] -> _
            shift-left: w603 -> [w609]
            shift-right: [w611] -> _
            shift-left: w604 -> [w614]
            tunnel: w603 -> [w608]
            stop <- w621 stop-if-true
            n153 = call "Bis zum nächsten Vielfachen warten3"("Count(mSec)"=u32 500) -> ()  [unwired: 1 out]
            n154 = global read "GVECDs.vi" "ECD1MW"() -> (w615:dbl[])
            n155 = global read "GVECDs.vi" "ECD2MW"() -> (w606:dbl[])
            n156 = Build Array (concatenate)(w616, w615) -> (w613:dbl[])
            n157 = Build Array (concatenate)(w609, w606) -> (w610:dbl[])
            n158 = global read "gvbooleschRT.vi" "global stop RT"() -> (w621:bool)
            n159 = global read "GVaktuelleTDMS.vi" "aktuelleTDMS-DateiECD1"() -> (w611:refnum<k34>)
            n160 = global read "GVaktuelleTDMS.vi" "aktuelleTDMS-DateiECD2"() -> (w619:refnum<k34>)
            n161 = Equal?(x=w614, y=w611) -> (x = y?=w607:bool)
            n162 = TDMS Write(0:w611, 7:"ECD1", 9:w615) -> ()  [unwired: 3 in, 4 out]
            n163 = TDMS Write(0:w619, 7:"ECD2", 9:w606) -> ()  [unwired: 3 in, 4 out]
            n164 = Select(t=w613, s=w607, f=w608) -> (s? t:f=w612:dbl[])
            n165 = Select(t=w610, s=w607, f=w608) -> (s? t:f=w605:dbl[])
            n166 = global write "GVChroms.vi" "ECD1Chrom"(w612) -> ()
            n167 = global write "GVChroms.vi" "ECD2Chrom"(w605) -> ()
          }
        }
      }
      n168 = while {
        shift-right: [w340] -> _
        shift-left: w234 -> [w342]
        shift-right: [w339] -> _
        shift-left: w234 -> [w341]
        stop <- w344 stop-if-true
        n169 = call "Bis zum nächsten Vielfachen warten"("Count(mSec)"=u32 100) -> ()  [unwired: 1 out]
        n170 = case shown="True" "An/Aus" {
          tunnel: w342 -> [w346 w362]
          tunnel: w341 -> [w345 w361]
          tunnel: [w346 w355] -> w340
          tunnel: [w345 w354] -> w339
          frame False {
          }
          frame True {
            w358 = dbl[] [] ("t")
            n171 = global read "GVMWHorst.vi" "MWHorst"() -> (w351:dbl[])
            n172 = global read "GVTrapsMachs.vi" "Traps/Machs"() -> (w352:dbl[])
            n173 = Build Array (concatenate)(w352, w351) -> (w350:dbl[])
            n174 = Index Array(array=w350, index="dargestellte Größe 3") -> (element=w363:dbl)
            n175 = Build Array (concatenate)(w362, w363) -> (w356:dbl[])
            n176 = Select(t=w358, s="TafelWischen!", f=w356) -> (s? t:f=w355:dbl[])
            n177 = global read "GVZeitenZyklen.vi" "Big Ben, Methodenzeit, Zykluszeit0, Zykluszeit1, Zykluszeit2A, Zykluszeit2B"() -> (w349:dbl[])
            n178 = Index Array(array=w349, index=1 ("Index")) -> (element=w347:dbl)
            n179 = Build Array (concatenate)(w361, w347) -> (w357:dbl[])
            n180 = Select(t=w358, s="TafelWischen!", f=w357) -> (s? t:f=w354:dbl[])
            n181 = Bundle(w357, w356) -> (→"schnelleAnzeige":cluster{dbl[], dbl[]})  [unwired: 1 in]
          }
        }
        n182 = global read "gvbooleschRT.vi" "global stop RT"() -> (w344:bool)
      }
      n183 = case shown="True" TRUE ("HKSpeichern") {
        tunnel: w331 -> [_ w644]
        frame False {
        }
        frame True {
          n184 = while {
            tunnel: w644 -> [w645]
            stop <- w661 stop-if-true
            n185 = call "Bis zum nächsten Vielfachen warten2"("Count(mSec)"=u32 1000) -> ()  [unwired: 1 out]
            n186 = global read "GVProbenvol.vi" "Probenvol.1"() -> (w648:dbl)
            n187 = global read "GVProbenvol.vi" "Probenvol.2"() -> (w647:dbl)
            n188 = global read "GVMWHorst.vi" "MWHorst"() -> (w656:dbl[])
            n189 = global read "GVZeitenZyklen.vi" "ZyklusNummern"() -> (w650:i32[])
            n190 = global read "gvbooleschRT.vi" "global stop RT"() -> (w661:bool)
            n191 = global read "GVZeitenZyklen.vi" "ZyklusNummernGesamt"() -> (w649:i32[])
            n192 = global read "GVaktuelleTDMS.vi" "aktuelleTDMS-DateiHK"() -> (w654:refnum<k34>)
            n193 = global read "GVHK1Hz.vi" "Mod1Mod2Mod3/AITrapsMachs1Hz"() -> (w655:dbl[])
            n194 = Index Array(array=w649, index=1 ("Index")) -> (element=w652:i32)
            n195 = To Double Precision Float(number=w652) -> (double precision float=w658:dbl)
            n196 = global read "GVZeitenZyklen.vi" "Big Ben, Methodenzeit, Zykluszeit0, Zykluszeit1, Zykluszeit2A, Zykluszeit2B"() -> (w651:dbl[])
            n197 = To Double Precision Float(number=w650) -> (double precision float=w657:dbl[])
            n198 = Build Array (concatenate)(w658, w657, w651, w655, w656, w648, w647) -> (w646:dbl[])
            n199 = TDMS Write(0:w654, 1:enum16{"decimated", "interleaved"}."interleaved" ("Daten-Layout (0:dezimiert)"), 7:w645, 9:w646) -> ()  [unwired: 2 in, 4 out]
          }
        }
      }
      n200 = for {
        N: 1 -> [_]
        tunnel: w260 -> [w673]
        tunnel: [w673] -> w287
        n201 = call "Warten8"("Count(mSec)"=u32 100) -> ()  [unwired: 1 out]
      }
      n202 = Build Array(w240) -> (w239:string[])
      n203 = Initialize Array(-1 ("Element"), 4 ("Dimension")) -> (w256:i32[])
      n204 = global read "GVVentilposition.vi" "Ventilposition"() -> (w266:i32)
      n205 = case shown="True" TRUE {
        tunnel: w282 -> [_ w628]
        tunnel: w280 -> [_ w627]
        tunnel: w279 -> [_ w626]
        tunnel: w274 -> [_ w625]
        tunnel: w273 -> [_ w624]
        frame False {
        }
        frame True {
          n206 = while {
            shift-right: [w629] -> w623
            shift-left: w625 -> [w631]
            shift-right: [w640] -> w622
            shift-left: w624 -> [w633]
            shift-right: [w635] -> _
            shift-left: w628 -> [w641]
            tunnel: w626 -> [w637]
            tunnel: w627 -> [w638]
            stop <- w643 stop-if-true
            n207 = call "Bis zum nächsten Vielfachen warten5"("Count(mSec)"=u32 500) -> ()  [unwired: 1 out]
            n208 = local read "Methode"() -> (w639:i32)
            n209 = global read "gvbooleschRT.vi" "global stop RT"() -> (w643:bool)
            n210 = global read "GVZeitenZyklen.vi" "ZyklusNummernGesamt"() -> (w630:i32[])
            n211 = Index Array(array=w630, index=1 ("Index")) -> (element=w635:i32)
            n212 = Greater?(x=w635, y=w641) -> (0:w634:bool)
            n213 = call "AktuelleTDMS.vi"("AktuelleTDMS"=w631, "Dateiordner"=w638, "NächsteTDMS"=w633, "NeuerZyklus?"=w634, "Methodennummer"=w639, "Zyklnumges"=w635, "Dateiname"=w637) -> ("AktuelleTDMS"=w629:refnum<k34>, "NächsteTDMS"=w640:refnum<k34>)  [unwired: 5 in, 2 out]
            n214 = Select(t=w633, s=w634, f=w631) -> (s? t:f=w632:refnum<k34>)
            n215 = global write "GVaktuelleTDMS.vi" "aktuelleTDMS-DateiHK"(w632) -> ()
          }
          n216 = TDMS Close(11:w623) -> ()  [unwired: 1 in, 2 out]
          n217 = TDMS Close(11:w622) -> ()  [unwired: 1 in, 2 out]
        }
      }
      n218 = case shown="True" TRUE {
        tunnel: w282 -> [_ w572]
        tunnel: w278 -> [_ w571]
        tunnel: w277 -> [_ w570]
        tunnel: w276 -> [_ w569]
        tunnel: w275 -> [_ w568]
        tunnel: w272 -> [_ w567]
        tunnel: w271 -> [_ w566]
        tunnel: w270 -> [_ w565]
        tunnel: w269 -> [_ w564]
        frame False {
        }
        frame True {
          n219 = while {
            shift-right: [w588] -> w563
            shift-left: w567 -> [w590]
            shift-right: [w598] -> w562
            shift-left: w566 -> [w592]
            shift-right: [w596] -> _
            shift-left: w572 -> [w599]
            tunnel: w571 -> [w595]
            tunnel: w569 -> [w594]
            stop <- w601 stop-if-true
            n220 = call "Bis zum nächsten Vielfachen warten4"("Count(mSec)"=u32 500) -> ()  [unwired: 1 out]
            n221 = local read "Methode"() -> (w597:i32)
            n222 = global read "gvbooleschRT.vi" "global stop RT"() -> (w601:bool)
            n223 = global read "GVZeitenZyklen.vi" "ZyklusNummernGesamt"() -> (w589:i32[])
            n224 = Index Array(array=w589, index=2 ("Index")) -> (element=w596:i32)
            n225 = Greater?(x=w596, y=w599) -> (0:w593:bool)
            n226 = call "AktuelleTDMS.vi"("AktuelleTDMS"=w590, "Dateiordner"=w595, "NächsteTDMS"=w592, "NeuerZyklus?"=w593, "Methodennummer"=w597, "Zyklnumges"=w596, "Dateiname"=w594) -> ("AktuelleTDMS"=w588:refnum<k34>, "NächsteTDMS"=w598:refnum<k34>)  [unwired: 5 in, 2 out]
            n227 = Select(t=w592, s=w593, f=w590) -> (s? t:f=w591:refnum<k34>)
            n228 = global write "GVaktuelleTDMS.vi" "aktuelleTDMS-DateiECD1"(w591) -> ()
          }
          n229 = while {
            shift-right: [w582] -> w561
            shift-left: w565 -> [w574]
            shift-right: [w583] -> w560
            shift-left: w564 -> [w576]
            shift-right: [w580] -> _
            shift-left: w572 -> [w584]
            tunnel: w570 -> [w579]
            tunnel: w568 -> [w578]
            stop <- w586 stop-if-true
            n230 = call "Bis zum nächsten Vielfachen warten6"("Count(mSec)"=u32 500) -> ()  [unwired: 1 out]
            n231 = local read "Methode"() -> (w581:i32)
            n232 = global read "gvbooleschRT.vi" "global stop RT"() -> (w586:bool)
            n233 = global read "GVZeitenZyklen.vi" "ZyklusNummernGesamt"() -> (w573:i32[])
            n234 = Index Array(array=w573, index=3 ("Index")) -> (element=w580:i32)
            n235 = Greater?(x=w580, y=w584) -> (0:w577:bool)
            n236 = call "AktuelleTDMS.vi"("AktuelleTDMS"=w574, "Dateiordner"=w579, "NächsteTDMS"=w576, "NeuerZyklus?"=w577, "Methodennummer"=w581, "Zyklnumges"=w580, "Dateiname"=w578) -> ("AktuelleTDMS"=w582:refnum<k34>, "NächsteTDMS"=w583:refnum<k34>)  [unwired: 5 in, 2 out]
            n237 = Select(t=w576, s=w577, f=w574) -> (s? t:f=w575:refnum<k34>)
            n238 = global write "GVaktuelleTDMS.vi" "aktuelleTDMS-DateiECD2"(w575) -> ()
          }
          n239 = TDMS Close(11:w563) -> ()  [unwired: 1 in, 2 out]
          n240 = TDMS Close(11:w562) -> ()  [unwired: 1 in, 2 out]
          n241 = TDMS Close(11:w561) -> ()  [unwired: 1 in, 2 out]
          n242 = TDMS Close(11:w560) -> ()  [unwired: 1 in, 2 out]
        }
      }
      n243 = Add(x=w298, y=w297) -> (x+y=w294:i32)
      n244 = Bundle(w239, w239, w239) -> (w305:cluster{string[], string[], string[]})  [unwired: 1 in]
      n245 = Index Array(array=w249, index=w247) -> (element=w248:T14)
      n246 = Initialize Array(cluster{"output high":dbl, "output low":dbl} {"output high"=99999.0, "output low"=0.0} ("output range"), w285) -> (w265:cluster{"output high":dbl, "output low":dbl}[])
      n247 = Concatenate Strings("?SE0,GDATA" ("Schreibpuffer"), "\r") -> (w235:string)
      n248 = Build Array(w296, w295, w294) -> (w293:i32[])
      n249 = while {
        tunnel: w332 -> [w801]
        shift-right: [w800] -> _
        shift-left: w249 -> [w778]
        tunnel: w265 -> [w799]
        tunnel: w264 -> [w798]
        tunnel: w260 -> [w797]
        tunnel: w263 -> [w796]
        tunnel: w262 -> [w795]
        shift-right: [w787] -> _
        shift-left: 0 -> [w794]
        tunnel: w260 -> [w793]
        tunnel: w259 -> [w792]
        shift-right: [w786] -> _
        shift-left: 0.0 -> [w791]
        shift-right: [w785] -> _
        shift-left: -1 -> [w790]
        shift-right: [w784] -> _
        shift-left: w256 -> [w789]
        tunnel: w255 -> [w779]
        tunnel: w254 -> [w780]
        tunnel: w253 -> [w781]
        tunnel: w252 -> [w782]
        tunnel: w251 -> [w783]
        tunnel: w250 -> [w788]
        shift-right: [w699] -> _
        shift-left: w248 -> [w698]
        tunnel: w233 -> [w677]
        tunnel: w232 -> [w681]
        tunnel: w231 -> [w687]
        i -> [w702]
        stop <- w802 stop-if-true
        w688 = 0  # ZeileMainMach2
        w689 = 0  # ZeileMainMach1
        w744 = FALSE
        w743 = 0.0
        w745 = 0  # ZeilennummerMPV
        w749 = cluster{dbl[], dbl[]} {[], []}
        w759 = dbl[] []
        w763 = 0  # ZeilePreMach2
        w764 = 0  # ZeilePreMach1
        w765 = 0  # ZeileFPGAFixp
        w766 = 0  # ZeileFPGAPID
        w767 = 0  # ZeileFPGABoolesch
        w768 = i32[] [0, 0, 0, 0]  # ZeilennummernHorst
        w769 = i32[] [0, 0, 0, 0]  # ZeilennummernDIOs
        n250 = Unbundle(w698) -> ("Zykluslängen [s]"=w742:dbl[], "ZeitpktDIOsMod0"=w741:dbl[], "ZeitpktDIOsMod1"=w740:dbl[], "ZeitpktDIOsMod2A"=w739:dbl[], "ZeitpktDIOsMod2B"=w738:dbl[], "DIOsSPMod0"=w737:bool[][], "DIOsSPMod1"=w736:bool[][], "DIOsSPMod2A"=w735:bool[][], "DIOsSPMod2B"=w734:bool[][], "Mod0HorstZeitpkt"=w733:dbl[], "Mod1HorstZeitpkt"=w732:dbl[], "Mod2AHorstZeitpkt"=w731:dbl[], "Mod2BHorstZeitpkt"=w730:dbl[], "HorstSPMod0"=w729:dbl[][], "HorstSPMod1"=w728:dbl[][], "HorstSPMod2A"=w727:dbl[][], "HorstSPMod2B"=w726:dbl[][], "LHSetpoints"=w725:dbl[], "LHHeizen?"=w724:bool[], "ZPktFPGABoolesch"=w723:dbl[], "FPGABoolesch"=w722:bool[][], "ZeitpktFPGAPID"=w721:dbl[], "FPGAPID"=w720:T17, "ZeitpktFPGAFixp"=w719:dbl[], "SHSetpoints"=w718:dbl[][], "t_PreMach1"=w717:dbl[], "T_PreMach1"=w716:dbl[], "t_PreMach2"=w715:dbl[], "T_PreMach2"=w714:dbl[], "PIDs für \"träge\" Heizungen"=w713:T18, "Zwangsbedingungen"=w712:dbl[][], "Dateien fürs MS schicken?"=w711:bool, "ZeitpunkteMPV"=w710:dbl[], "SPMPV"=w709:i32[], "ZeitpktMS-1"=w708:dbl, "ZeitpktMS-2"=w707:dbl, "Int.Start1"=w706:dbl, "Int.Stop1"=w705:dbl, "Int.Start2"=w704:dbl, "Int.Stop2"=w703:dbl, "t_MainMach1"=w697:dbl[], "T_MainMach1"=w696:dbl[], "t_MainMach2"=w695:dbl[], "T_MainMach2"=w694:dbl[])  [unwired: 1 out]
        "Zykluslängen [s]" <- w742
        n251 = Add(x=w789, y=1) -> (x+y=w753:i32[])
        n252 = Add(x=w790, y=1) -> (x+y=w775:i32)
        n253 = Array Subset(array=w687, index=2 ("Index"), length=4 ("Länge")) -> (w684:dbl[])
        n254 = Array Subset(array=w681, index=2 ("Index"), length=4 ("Länge")) -> (w680:dbl[])
        n255 = Array Subset(array=w677, index=2 ("Index"), length=4 ("Länge")) -> (w676:dbl[])
        n256 = local read "Methode"() -> (w701:i32)
        n257 = while {
          tunnel: w780 -> [w954]
          tunnel: w783 -> [w952]
          tunnel: w782 -> [w951]
          tunnel: w779 -> [w953]
          tunnel: w781 -> [w950]
          tunnel: w712 -> [w942]
          stop <- w944 stop-if-true
          n258 = call "Bis zum nächsten Vielfachen warten10"("Count(mSec)"=u32 1000) -> ()  [unwired: 1 out]
          n259 = local read "Methode"() -> (w949:i32)
          n260 = global read "GVMethodenwechsel.vi" "Methodenwechsel?"() -> (w946:bool)
          n261 = global read "gvbooleschRT.vi" "global stop RT"() -> (w947:bool)
          n262 = case shown="True" "global stop RT" {
            frame False {
            }
            frame True {
              n263 = global write "gvbooleschRT.vi" "global stop RT"(TRUE ("global stop RT")) -> ()
            }
          }
          n264 = call "ZwangsbedingungenGV.vi"("AnzahlHorst"=w952, "AnzahlHorst/Modul"=w953, "AnzahlLH"=w951, "AnzahlDIOs/Modul"=w954, "AnzahlDIOs"=w950, "Zwangsbedingungen"=w942, "Methodennummer"=w949) -> ("Methodennummer"=w948:i32)  [unwired: 4 in]
          n265 = local write "Methode"(w948) -> ()
          n266 = local read "veränderte Methode benutzen"() -> (w945:bool)
          n267 = Compound Arithmetic op=OR(w947, w946, w945) -> (w944:bool)
        }
        n268 = while {
          tunnel: w798 -> [w865]
          tunnel: w799 -> [w866]
          tunnel: w797 -> [w862]
          tunnel: w725 -> [w856]
          tunnel: w713 -> [w855]
          stop <- w851 stop-if-true
          n269 = global read "GVAIs.vi" "AIs"() -> (w857:dbl[])
          n270 = call "Bis zum nächsten Vielfachen warten12"("Count(mSec)"=u32 100) -> ()  [unwired: 1 out]
          n271 = global read "GVHeizenLH.vi" "Heizen?LH"() -> (w858:bool[])
          n272 = for {
            tunnel: w857 -> [w941]
            tunnel: w865 -> [w940] mode=indexing
            tunnel: [w939] -> w864 mode=indexing
            n273 = Index Array(array=w941, index=w940) -> (element=w939:dbl)
          }
          n274 = global read "GVMethodenwechsel.vi" "Methodenwechsel?"() -> (w853:bool)
          n275 = global read "gvbooleschRT.vi" "global stop RT"() -> (w854:bool)
          n276 = Array To Cluster(array=w858) -> (cluster=w861:T19)
          n277 = local read "veränderte Methode benutzen"() -> (w852:bool)
          n278 = call-poly <vilib>:"PID.vi"("output range"=w866, "PID gains"=w855, "process variable"=w864, "setpoint"=w856) -> ("output"=w863:dbl[])  [unwired: 6 in, 1 out]
          n279 = Compound Arithmetic op=OR(w854, w853, w852) -> (w851:bool)
          n280 = To Unsigned Long Integer(number=w863) -> (unsigned 32bit integer=w860:u32[])
          n281 = Array To Cluster(array=w860) -> (cluster=w859:T20)
          n282 = xnode "Read/Write Control"("FPGA VI Reference In"=w862, "LHHeizen?"=w861, "LHPulse(us)"=w859) -> ()  [unwired: 1 in, 2 out]
        }
        n283 = Build Cluster Array(w737, w736, w735, w734) -> (w773:cluster{"DIOsSPMod2B":bool[][]}[])
        n284 = Build Cluster Array(w729, w728, w727, w726) -> (w771:cluster{"HorstSPMod2B":dbl[][]}[])
        n285 = Build Cluster Array(w741, w740, w739, w738) -> (w774:cluster{"ZeitpktDIOsMod2B":dbl[]}[])
        n286 = Build Cluster Array(w733, w732, w731, w730) -> (w772:cluster{"Mod2BHorstZeitpkt":dbl[]}[])
        n287 = Bundle(w684, w680, w676) -> (w675:cluster{dbl[], dbl[], dbl[]})  [unwired: 1 in]
        n288 = Equal?(x=w702, y=0) -> (x = y?=w776:bool)
        n289 = global read "GVZeitenZyklen.vi" "ZyklusNummern"() -> (w752:i32[])
        n290 = global read "GVZwangs.vi" "ZwangsHorst?"() -> (w758:cluster{bool[]}[])
        n291 = global read "gvbooleschRT.vi" "global stop RT"() -> (w802:bool)
        n292 = global read "GVZwangs.vi" "ZwangsDIO?"() -> (w757:cluster{bool[]}[])
        n293 = while {
          shift-right: [w815] -> _
          shift-left: w744 -> [w819]
          shift-right: [w814] -> _
          shift-left: w743 -> [w818]
          shift-right: [w813] -> _
          shift-left: w744 -> [w817]
          shift-right: [w812] -> _
          shift-left: w743 -> [w816]
          tunnel: w788 -> [w811]
          tunnel: w706 -> [w806]
          tunnel: w705 -> [w805]
          tunnel: w704 -> [w804]
          tunnel: w703 -> [w803]
          stop <- w808 stop-if-true
          n294 = call "Integrieren.vi"("Integrieren1"=w819, "Integral1"=w818, "Integrieren2"=w817, "Integral2"=w816, "Int.Start1"=w806, "Int.Stop1"=w805, "Int.Start2"=w804, "HorstProbenflußNr."=w811, "Int.Stop2"=w803) -> ("Integrieren1"=w815:bool, "Integral1"=w814:dbl, "Integrieren2"=w813:bool, "Integral2"=w812:dbl)  [unwired: 7 in]
          n295 = call "Bis zum nächsten Vielfachen warten9"("Count(mSec)"=u32 100) -> ()  [unwired: 1 out]
          n296 = global read "GVMethodenwechsel.vi" "Methodenwechsel?"() -> (w809:bool)
          n297 = global read "gvbooleschRT.vi" "global stop RT"() -> (w810:bool)
          n298 = local read "veränderte Methode benutzen"() -> (w807:bool)
          n299 = Compound Arithmetic op=OR(w810, w809, w807) -> (w808:bool)
        }
        n300 = while "Zeit" {
          tunnel: w776 -> [w1088]
          tunnel: [w1083] -> w786
          tunnel: w791 -> [w1087]
          tunnel: [w1077] -> w785
          tunnel: w775 -> [w1078]
          tunnel: w742 -> [w1085]
          tunnel: w753 -> [w1072]
          tunnel: [w1069] -> w784
          i -> [w1091]
          stop <- w1074 stop-if-true
          n301 = Equal?(x=w1091, y=0) -> (x = y?=w1089:bool)
          n302 = call "Bis zum nächsten Vielfachen warten15"("Count(mSec)"=u32 50) -> ()  [unwired: 1 out]
          n303 = And(x=w1088, y=w1089) -> (x .and. y?=w1093:bool)
          n304 = xnode "Elapsed Timer"("reset"=w1093) -> ("elapsed time (ms)"=w1096:i32)  [unwired: 2 in, 1 out]
          n305 = global read "GVMethodenwechsel.vi" "Methodenwechsel?"() -> (w1073:bool)
          n306 = global read "gvbooleschRT.vi" "global stop RT"() -> (w1086:bool)
          n307 = local read "veränderte Methode benutzen"() -> (w1076:bool)
          n308 = Or(x=w1073, y=w1086) -> (x .or. y?=w1075:bool)
          n309 = To Double Precision Float(number=w1096) -> (double precision float=w1095:dbl)
          n310 = Divide(x=w1095, y=1000.0) -> (x/y=w1083:dbl)
          n311 = Or(x=w1076, y=w1075) -> (x .or. y?=w1074:bool)
          n312 = Subtract(x=w1083, y=w1087) -> (x-y=w1082:dbl)
          n313 = for {
            tunnel: w1085 -> [w1099] mode=indexing
            tunnel: w1082 -> [w1100]
            tunnel: [w1098] -> w1084 mode=indexing
            tunnel: [w1097] -> w1081 mode=indexing
            n314 = Quotient & Remainder(x=w1100, y=w1099) -> (x-y*floor(x/y)=w1098:dbl, floor(x/y)=w1097:dbl)
          }
          n315 = Build Array (concatenate)(w1083, w1082, w1084) -> (w1071:dbl[])
          n316 = To Long Integer(number=w1081) -> (32bit integer=w1070:i32[])
          n317 = global write "GVZeitenZyklen.vi" "ZyklusNummern"(w1070) -> ()
          n318 = global write "GVZeitenZyklen.vi" "Big Ben, Methodenzeit, Zykluszeit0, Zykluszeit1, Zykluszeit2A, Zykluszeit2B"(w1071) -> ()
          n319 = Add(x=w1070, y=w1072) -> (x+y=w1069:i32[])
          n320 = Index Array(array=w1070, index=1 ("Index")) -> (element=w1079:i32)
          n321 = global write "GVZeitenZyklen.vi" "ZyklusNummernGesamt"(w1069) -> ()
          n322 = Add(x=w1079, y=w1078) -> (x+y=w1077:i32)
        }
        n323 = Bundle(w774, w773, w772, w771, "LHHeizen?"=w724, "ZPktFPGABoolesch"=w723, "FPGABoolesch"=w722, "ZeitpktFPGAPID"=w721, "FPGAPID"=w720, "ZeitpktFPGAFixp"=w719, "SHSetpoints"=w718, "t_PreMach1"=w717, "T_PreMach1"=w716, "t_PreMach2"=w715, "T_PreMach2"=w714, "ZeitpunkteMPV"=w710, "SPMPV"=w709, "t_MainMach1"=w697, "T_MainMach1"=w696, "t_MainMach2"=w695, "T_MainMach2"=w694) -> (w770:T21)  [unwired: 1 in]
        n324 = global read "GVaktuelleTDMS.vi" "aktuelleTDMS-DateiECD1"() -> (w751:refnum<k34>)
        n325 = Index Array(array=w778, index=w701) -> (element=w700:T14)
        n326 = global read "GVZwangs.vi" "ZwangsFPGABoolesch?"() -> (w756:bool[])
        n327 = while {
          tunnel: w801 -> [w1150]
          shift-right: [w1141] -> _
          shift-left: w700 -> [w1149]
          tunnel: w701 -> [w1147]
          shift-right: [w1139] -> w800
          shift-left: w778 -> [w1148]
          tunnel: [w1140] -> w699
          stop <- w1143 stop-if-true
          n328 = call "Bis zum nächsten Vielfachen warten8"("Count(mSec)"=u32 500) -> ()  [unwired: 1 out]
          n329 = global read "GVMethodenwechsel.vi" "Methodenwechsel?"() -> (w1145:bool)
          n330 = global read "gvbooleschRT.vi" "global stop RT"() -> (w1144:bool)
          n331 = case shown="True" "Methode verändern" {
            tunnel: w1150 -> [_ w1172]
            tunnel: w1149 -> [w1169 w1171]
            tunnel: [w1169 w1170] -> w1141
            frame False {
            }
            frame True {
              n332 = call "methodeändern-11-15.vi"("Methode"=w1171, "Namen"=w1172) -> ("Methode"=w1170:T22)  [unwired: 1 in]
              n333 = property on="Methode verändern" class="Bool (strict)"("Value"=FALSE ("Methode verändern")) -> ()  [unwired: 2 in, 2 out]
            }
          }
          n334 = Compound Arithmetic op=OR(w1145, w1144, "veränderte Methode benutzen") -> (w1143:bool)
          n335 = case shown="True" "Methode speichern" {
            tunnel: w1141 -> [_ w1166]
            tunnel: w1148 -> [w1159 w1168]
            tunnel: w1147 -> [_ w1167]
            tunnel: [w1159 w1161] -> w1139
            frame False {
            }
            frame True {
              n336 = Replace Array Subset(array=w1168, new element=w1166, index=w1167) -> (w1161:T7)
              n337 = property on="Methode speichern" class="Bool (strict)"("Value"=FALSE ("Methode speichern")) -> ()  [unwired: 2 in, 2 out]
              n338 = Open/Create/Replace File(file path (use dialog)=path "c:/methoden.per" ("Dateipfad (Dialog verwenden)"), operation (0:open)=T9."replace" ("Operation (0:Öffnen)")) -> (refnum out=w1163:refnum<file>)  [unwired: 4 in, 2 out]
              n339 = Write to Binary File(file (use dialog)=w1163, data=w1161) -> (refnum out=w1160:refnum<file>)  [unwired: 4 in, 2 out]
              n340 = Close File(refnum=w1160) -> ()  [unwired: 1 in, 2 out]
            }
          }
          n341 = case shown="False" "veränderte Methode benutzen" {
            tunnel: w1141 -> [_ w1156]
            tunnel: [w1153 w1156] -> w1140
            tunnel: w1139 -> [w1155 _]
            frame False {
              n342 = local read "Methode"() -> (w1154:i32)
              n343 = Index Array(array=w1155, index=w1154) -> (element=w1153:T14)
            }
            frame True {
              n344 = flat-sequence {
                frame #0 {
                  n345 = call "Warten"("Count(mSec)"=u32 1100) -> ()  [unwired: 1 out]
                }
                frame #1 {
                  n346 = property on="veränderte Methode benutzen" class="Bool (strict)"("Value"=FALSE ("Methode verändern")) -> ()  [unwired: 2 in, 2 out]
                }
              }
            }
          }
        }
        n347 = Bundle(w759, w759, w759, w759) -> (w760:cluster{dbl[], dbl[], dbl[], dbl[]})  [unwired: 1 in]
        n348 = Bundle("ZyklusNummern"=w752, "ZeilennummernDIOs"=w769, "ZwangsDIO?"=w757, "ZeilennummernHorst"=w768, "ZwangsHorst?"=w758, "ZeileFPGABoolesch"=w767, "ZwangsFPGABoolesch?"=w756, "ZeileFPGAPID"=w766, "ZeileFPGAFixp"=w765, "ZeilePreMach1"=w764, "ZeilePreMach2"=w763, "ZeilennummerMPV"=w745, "ZeileMainMach1"=w689, "ZeileMainMach2"=w688) -> (w762:T23)  [unwired: 1 in]
        n349 = call "arrayDoppelMoppel-11-15.vi"("verdoppeln"=i32[] [0, 1], "Traps/MachsKoeff2"=w677, "Traps/MachsKoeff1"=w681, "Traps/MachsKoeff0"=w687) -> ("Traps/MachsKoeff2"=w690:dbl[], "Traps/MachsKoeff1"=w691:dbl[], "Traps/MachsKoeff0"=w692:dbl[])  [unwired: 5 in]
        n350 = while "ZyklusSteuerung" {
          tunnel: w792 -> [w1067]
          tunnel: w793 -> [w1060]
          shift-right: [w1056] -> _
          shift-left: w762 -> [w1065]
          tunnel: w770 -> [w1066]
          tunnel: w692 -> [w1059]
          tunnel: w691 -> [w1058]
          tunnel: w690 -> [w1057]
          tunnel: w675 -> [w1055]
          stop <- w1061 stop-if-true
          n351 = call "ZyklussteuerungGV-11-15.vi"("MachKoeffs"=w1055, "FPGA VI Reference In"=w1060, "Zeitpunkte/Setpoints"=w1066, "DIOsNummern"=w1067, "Schieberegister"=w1065, "Traps/MachKoeff2"=w1057, "Traps/MachKoeff1"=w1058, "Traps/MachKoeff0"=w1059) -> ("Schieberegister"=w1056:T24)  [unwired: 3 in]
          n352 = call "Bis zum nächsten Vielfachen warten11"("Count(mSec)"=u32 100) -> ()  [unwired: 1 out]
          n353 = global read "GVMethodenwechsel.vi" "Methodenwechsel?"() -> (w1064:bool)
          n354 = global read "gvbooleschRT.vi" "global stop RT"() -> (w1063:bool)
          n355 = local read "veränderte Methode benutzen"() -> (w1062:bool)
          n356 = Compound Arithmetic op=OR(w1064, w1063, w1062) -> (w1061:bool)
        }
        n357 = while {
          shift-right: [w1003] -> _
          shift-left: w760 -> [w1010]
          shift-right: [w1002] -> _
          shift-left: w760 -> [w1009]
          shift-right: [w1000] -> _
          shift-left: T13 {"Zyklus1"=0, "Zeitachse1"=0, "dargestellte Größe 1"=0, "Zyklus2"=0, "Zeitachse2"=0, "dargestellte Größe 2"=0} ("AnzeigeEinstellungen") -> [w1008]
          tunnel: w742 -> [w978]
          shift-right: [w974] -> _
          shift-left: w751 -> [w973]
          shift-right: [w969] -> _
          shift-left: w749 -> [w971]
          shift-right: [w958] -> _
          shift-left: w749 -> [w970]
          shift-right: ["Detektor"] -> _
          shift-left: 0 ("Detektor") -> [w967]
          stop <- w1014 stop-if-true
          w979 = 0.0 ("X-Achse.Bereich:Minimum")
          n358 = call "Bis zum nächsten Vielfachen warten14"("Count(mSec)"=u32 1000) -> ()  [unwired: 1 out]
          n359 = case shown="True" TRUE ("Tabellarische Darstellung") {
            frame False {
            }
            frame True {
              n360 = global read "GVHK1Hz.vi" "Mod1Mod2Mod3/AITrapsMachs1Hz"() -> (w1020:dbl[])
              n361 = Array Subset(array=w1020, index=0 ("Index"), length=32 ("Länge")) -> (→"AIs1":dbl[])
              n362 = Array Subset(array=w1020, index=32 ("Index"), length=32 ("Länge")) -> (→"AIs2":dbl[])
              n363 = Array Subset(array=w1020, index=64 ("Index"), length=32 ("Länge")) -> (→"AIs3":dbl[])
            }
          }
          n364 = case shown="0, Default" "Detektor" {
            tunnel: [w1034 w1046] -> w969
            tunnel: w978 -> [w1033 w1048]
            tunnel: "Detektor" -> [w1028 w1042]
            tunnel: [w1032 w1047] -> w976
            tunnel: [w1031 w1045] -> w974
            frame 0, Default {
              n365 = Increment(x=w1028) -> (x+1=w1029:i32)
              n366 = Increment(x=w1029) -> (x+1=w1027:i32)
              n367 = global read "GVChroms.vi" "ECD1Chrom"() -> (w1030:dbl[])
              n368 = global read "GVaktuelleTDMS.vi" "aktuelleTDMS-DateiECD1"() -> (w1031:refnum<k34>)
              n369 = Index Array(array=w1033, index=w1027) -> (element=w1032:dbl)
              n370 = Array Size(array=w1030) -> (size(s)=w1036:i32)
              n371 = for {
                N: w1036 -> [_]
                tunnel: [w1037] -> w1035 mode=indexing
                i -> [w1040]
                n372 = To Double Precision Float(number=w1040) -> (double precision float=w1039:dbl)
                n373 = Divide(x=w1039, y=10.0) -> (x/y=w1037:dbl)
              }
              n374 = Bundle(w1035, "ECD1Chrom"=w1030) -> (w1034:cluster{dbl[], "ECD1Chrom":dbl[]})  [unwired: 1 in]
            }
            frame 1 {
              n375 = Increment(x=w1042) -> (x+1=w1043:i32)
              n376 = Increment(x=w1043) -> (x+1=w1041:i32)
              n377 = global read "GVChroms.vi" "ECD2Chrom"() -> (w1044:dbl[])
              n378 = global read "GVaktuelleTDMS.vi" "aktuelleTDMS-DateiECD2"() -> (w1045:refnum<k34>)
              n379 = Index Array(array=w1048, index=w1041) -> (element=w1047:dbl)
              n380 = Array Size(array=w1044) -> (size(s)=w1050:i32)
              n381 = for {
                N: w1050 -> [_]
                tunnel: [w1051] -> w1049 mode=indexing
                i -> [w1054]
                n382 = To Double Precision Float(number=w1054) -> (double precision float=w1053:dbl)
                n383 = Divide(x=w1053, y=10.0) -> (x/y=w1051:dbl)
              }
              n384 = Bundle(w1049, "ECD2Chrom"=w1044) -> (w1046:cluster{dbl[], "ECD2Chrom":dbl[]})  [unwired: 1 in]
            }
          }
          n385 = Equal?(x="Detektor", y=w967) -> (x = y?=w966:bool)
          n386 = Subtract(x="DetYMax", y="DetYMin") -> (x-y=w984:dbl)
          n387 = Subtract(x="HK2YMax", y="HK2YMin") -> (x-y=w989:dbl)
          n388 = Subtract(x="HK1YMax", y="HK1YMin") -> (x-y=w994:dbl)
          n389 = global read "GVMethodenwechsel.vi" "Methodenwechsel?"() -> (w1012:bool)
          n390 = global read "GVZeitenZyklen.vi" "ZyklusNummern"() -> (w981:i32[])
          "ZyklusNummern" <- w981
          n391 = global read "gvbooleschRT.vi" "global stop RT"() -> (w1013:bool)
          n392 = Divide(x=w984, y=20.0) -> (x/y=w982:dbl)
          n393 = Divide(x=w989, y=10.0) -> (x/y=w987:dbl)
          n394 = Divide(x=w994, y=10.0) -> (x/y=w992:dbl)
          n395 = global read "GVZeitenZyklen.vi" "ZyklusNummernGesamt"() -> (→"ZyklusNummernGesamt":i32[])
          n396 = local read "veränderte Methode benutzen"() -> (w1011:bool)
          n397 = Or(x=w1012, y=w1013) -> (x .or. y?=w1015:bool)
          n398 = Or(x=w1015, y=w1011) -> (x .or. y?=w1014:bool)
          n399 = global read "GVZeitenZyklen.vi" "Big Ben, Methodenzeit, Zykluszeit0, Zykluszeit1, Zykluszeit2A, Zykluszeit2B"() -> (w961:dbl[])
          n400 = To Long Integer(number=w961) -> (32bit integer=→"Big Ben, Methodenzeit, Zykluszeit0, Zykluszeit1, Zykluszeit2A, Zykluszeit2B":i32[])
          n401 = Equal?(x=w974, y=w973) -> (x = y?=w972:bool)
          n402 = call "AnzeigeGV.vi"("veränderte Methode benutzen"=w1011, "Zykluslängen [s]"=w978, "Cluster1"=w1010, "Big Ben, Methodenzeit, Zykluszeit0, Zykluszeit1, Zykluszeit2A, Zykluszeit2B"=w961, "Zyklusnummern 0, 1, 2A, 2B"=w981, "Cluster2"=w1009, "AnzeigeEinstellungen"=w1008, "dargestellte Größe 1"="dargestellte Größe 1", "Zeitachse1"="Zeitachse1", "dargestellte Größe 2"="dargestellte Größe 2", "Zeitachse2"="Zeitachse2") -> ("Anzeige2"=→"Housekeeping2":cluster{dbl[], dbl[]}, "Cluster1"=w1003:cluster{dbl[], dbl[], dbl[], dbl[]}, "x1Inkr"=w998:dbl, "Cluster2"=w1002:cluster{dbl[], dbl[], dbl[], dbl[]}, "Anzeige1"=→"Housekeeping1":cluster{dbl[], dbl[]}, "AnzeigeEinstellungen"=w1000:T13, "x2Max"=w962:dbl, "x2Inkr"=w997:dbl, "x1Max"=w963:dbl)  [unwired: 8 in]
          n403 = Divide(x=w976, y=20.0) -> (x/y=w977:dbl)
          n404 = Select(t=w970, s=w972, f=w971) -> (s? t:f=w965:cluster{dbl[], dbl[]})
          n405 = property on="Detektor 2" class="XYGraph (strict)"("XScale.Minimum"=w979, "XScale.Maximum"=w976, "XScale.Increment"=w977, "YScale.Minimum"="DetYMin", "YScale.Maximum"="DetYMax", "YScale.Increment"=w982) -> ()  [unwired: 2 in, 2 out]
          n406 = property on="Housekeeping2" class="XYGraph (strict)"("XScale.Minimum"=w979, "XScale.Maximum"=w962, "XScale.Increment"=w997, "YScale.Minimum"="HK2YMin", "YScale.Maximum"="HK2YMax", "YScale.Increment"=w987) -> ()  [unwired: 2 in, 2 out]
          n407 = property on="Housekeeping1" class="XYGraph (strict)"("XScale.Minimum"=w979, "XScale.Maximum"=w963, "XScale.Increment"=w998, "YScale.Minimum"="HK1YMin", "YScale.Maximum"="HK1YMax", "YScale.Increment"=w992) -> ()  [unwired: 2 in, 2 out]
          n408 = Select(t=w965, s=w966, f=cluster{dbl[], dbl[]} {[], []} ("s? t:f")) -> (s? t:f=w958:cluster{dbl[], dbl[]})
          n409 = Build Array(w969, w958) -> (→"Detektor 2":cluster{dbl[], "ECD2Chrom":dbl[]}[])
        }
        n410 = global read "GVZeitenZyklen.vi" "Big Ben, Methodenzeit, Zykluszeit0, Zykluszeit1, Zykluszeit2A, Zykluszeit2B"() -> (w748:dbl[])
        n411 = Index Array(array=w748, index=3 ("Index")) -> (element=w746:dbl)
        n412 = while {
          tunnel: w796 -> [w823]
          tunnel: w795 -> [w822]
          tunnel: w711 -> [w837]
          shift-right: [w838] -> w787
          shift-left: w794 -> [w839]
          tunnel: w708 -> [w833]
          tunnel: w707 -> [w827]
          shift-right: [w824] -> _
          shift-left: w746 -> [w828]
          stop <- w840 stop-if-true
          n413 = Less?(x=w828, y=w827) -> (x < y?=w829:bool)
          n414 = Less?(x=w828, y=w833) -> (x < y?=w831:bool)
          n415 = call "Bis zum nächsten Vielfachen warten13"("Count(mSec)"=u32 100 ("Zu wartende ms")) -> ()  [unwired: 1 out]
          n416 = global read "GVMethodenwechsel.vi" "Methodenwechsel?"() -> (w842:bool)
          n417 = global read "gvbooleschRT.vi" "global stop RT"() -> (w843:bool)
          n418 = local read "veränderte Methode benutzen"() -> (w841:bool)
          n419 = Compound Arithmetic op=OR(w843, w842, w841) -> (w840:bool)
          n420 = global read "GVZeitenZyklen.vi" "Big Ben, Methodenzeit, Zykluszeit0, Zykluszeit1, Zykluszeit2A, Zykluszeit2B"() -> (w835:dbl[])
          n421 = Index Array(array=w835, index=3 ("Index")) -> (element=w824:dbl)
          n422 = Greater Or Equal?(x=w824, y=w827) -> (x >= y?=w830:bool)
          n423 = Greater Or Equal?(x=w824, y=w833) -> (x >= y?=w832:bool)
          n424 = And(x=w830, y=w829) -> (x .and. y?=w826:bool)
          n425 = And(x=w832, y=w831) -> (x .and. y?=w821:bool)
          n426 = Or(x=w821, y=w826) -> (x .or. y?=w825:bool)
          n427 = And(x=w837, y=w825) -> (x .and. y?=w836:bool)
          n428 = case shown="True" w836 {
            tunnel: w839 -> [w845 w846]
            tunnel: [w845 w850] -> w838
            tunnel: w823 -> [_ w849]
            tunnel: w822 -> [_ w848]
            tunnel: w821 -> [_ w847]
            frame False {
            }
            frame True {
              n429 = call "MSDateienSchicken12-15.vi"("MSNummer"=w846, "MSa?"=w847, "Dateipfad:fromcriordy"=w848, "Dateipfad:fromcriocmd"=w849) -> ()  [unwired: 1 in]
              n430 = Increment(x=w846) -> (x+1=w850:i32)
            }
          }
        }
      }
      n431 = Add Array Elements(numeric array=w293) -> (sum=w303:i32)
      n432 = Index Array(array=w293, index #1=0 ("Index"), index #2=1 ("Index")) -> (element #1=w314:i32, element #2=w312:i32)
      n433 = Split 1D Array(array=w292, index=w314) -> (first subarray=w318:dbl[], second subarray=w322:dbl[])
      n434 = Split 1D Array(array=w290, index=w314) -> (first subarray=w321:string[], second subarray=w323:string[])
      n435 = Split 1D Array(array=w291, index=w314) -> (first subarray=w311:string[], second subarray=w313:string[])
      n436 = Initialize Array(-1.0 ("Element"), w303) -> (w288:dbl[])
      n437 = Split 1D Array(array=w323, index=w312) -> (first subarray=w320:string[], second subarray=w319:string[])
      n438 = Split 1D Array(array=w322, index=w312) -> (first subarray=w317:dbl[], second subarray=w316:dbl[])
      n439 = Split 1D Array(array=w313, index=w312) -> (first subarray=w310:string[], second subarray=w309:string[])
      n440 = Bundle(w321, w320, w319, w318, w317, w316) -> (w315:T25)  [unwired: 1 in]
      n441 = Bundle(w311, w310, w309) -> (w308:cluster{string[], string[], string[]})  [unwired: 1 in]
      n442 = Bundle(w307, w307, w307) -> (w306:cluster{i32, i32, i32})  [unwired: 1 in]
      n443 = Initialize Array(0.0, 8 ("Dimension")) -> (w236:dbl[])
      n444 = Initialize Array("x", 8 ("Dimension")) -> (w241:string[])
      n445 = case shown="True" TRUE ("SerielleKomm.") {
        tunnel: bool[] [TRUE, TRUE, TRUE, TRUE, TRUE, TRUE, TRUE, TRUE] -> [_ w378]
        tunnel: w241 -> [_ w377]
        tunnel: w315 -> [_ w376]
        tunnel: w314 -> [_ w375]
        tunnel: w312 -> [_ w374]
        tunnel: w308 -> [_ w373]
        tunnel: w306 -> [_ w372]
        tunnel: w305 -> [_ w371]
        tunnel: w292 -> [_ w370]
        tunnel: w289 -> [_ w369]
        tunnel: w288 -> [_ w368]
        tunnel: w287 -> [_ w365]
        tunnel: w266 -> [_ w367]
        tunnel: w236 -> [_ w366]
        tunnel: w235 -> [_ w364]
        frame False {
        }
        frame True {
          n446 = while {
            tunnel: w365 -> [w386]
            tunnel: w364 -> [w385]
            stop <- w388 stop-if-true
            n447 = String To Byte Array(string=w385) -> (unsigned byte array=w381:u8[])
            n448 = call "Warten6"("Count(mSec)"=u32 500) -> ()  [unwired: 1 out]
            n449 = Join Numbers(hi=w381, lo=u8 5) -> ((hi.lo)=w383:u16[])
            n450 = Join Numbers(hi=w381, lo=u8 6) -> ((hi.lo)=w379:u16[])
            n451 = xnode "Invoke Method"("FPGA VI Reference In"=w386, "Data"=w383) -> ("FPGA VI Reference Out"=w382:refnum<k20>)  [unwired: 2 in, 2 out]
            n452 = global read "gvbooleschRT.vi" "global stop RT"() -> (w388:bool)
            n453 = xnode "Invoke Method"("FPGA VI Reference In"=w382, "Data"=w379) -> ()  [unwired: 2 in, 3 out]
          }
          n454 = while {
            shift-right: [w548] -> _
            shift-left: w378 -> [w523]
            shift-right: [w531] -> _
            shift-left: w368 -> [w543]
            tunnel: w365 -> [w530]
            shift-right: [w521] -> _
            shift-left: w377 -> [w547]
            tunnel: w369 -> [w546]
            tunnel: w370 -> [w545]
            shift-right: [w533] -> _
            shift-left: w371 -> [w535]
            tunnel: w375 -> [w541]
            tunnel: w374 -> [w542]
            tunnel: w376 -> [w544]
            tunnel: w373 -> [w538]
            shift-right: [w537] -> _
            shift-left: w372 -> [w539]
            shift-right: [w527] -> _
            shift-left: w367 -> [w529]
            shift-right: [w524] -> _
            shift-left: w366 -> [w525]
            stop <- w532 stop-if-true
            n455 = for {
              tunnel: w523 -> [w552] mode=indexing
              tunnel: w525 -> [w549] mode=indexing
              tunnel: [w556] -> w524 mode=indexing
              tunnel: [w553] -> w522 mode=indexing
              n456 = global read "GVZeitenZyklen.vi" "Big Ben, Methodenzeit, Zykluszeit0, Zykluszeit1, Zykluszeit2A, Zykluszeit2B"() -> (w559:dbl[])
              n457 = Index Array(array=w559, index=0 ("Index")) -> (element=w557:dbl)
              n458 = Subtract(x=w557, y=w549) -> (x-y=w555:dbl)
              n459 = Greater?(x=w555, y=0.1) -> (0:w551:bool)
              n460 = Or(x=w552, y=w551) -> (x .or. y?=w550:bool)
              n461 = Select(t=w551, s=w551, f=w552) -> (s? t:f=w553:bool)
              n462 = Select(t=w557, s=w550, f=w549) -> (s? t:f=w556:dbl)
            }
            n463 = call "MPVSenden-11-15.vi"("Ventilposition"=w529, "FPGA VI Reference In"=w530) -> ("Ventilposition"=w527:i32, "FPGA VI Reference Out"=w528:refnum<k20>)
            n464 = call "Warten3"("Count(mSec)"=u32 10) -> ()  [unwired: 1 out]
            n465 = global read "GVHorstSP.vi" "HorstSP"() -> (w531:dbl[])
            n466 = Not Equal?(x=w531, y=w543) -> (x != y?=w536:bool)
            n467 = global read "gvbooleschRT.vi" "global stop RT"() -> (w532:bool)
            n468 = call "NeueSP.vi"("Anzahl2"=w542, "Anzahl1"=w541, "AlteSP"=w543, 7:"NeueSP"=w531, "BefehleCluster"=w535, 10:"NeueSP"=w536, "ClusterFest"=w544) -> ("BefehleCluster"=w534:T26)  [unwired: 4 in]
            n469 = call "Senden-11-15.vi"("FPGA VI Reference In"=w528, "BefehlsCluster"=w534, "Senden?"=w522, "Abfragenr.Cluster"=w539, "AbfragenCluster"=w538) -> ("Senden?"=w540:bool[], "Abfragenr.Cluster"=w537:cluster{i32, i32, i32}, "BefehlsCluster"=w533:T26)  [unwired: 1 in]
            n470 = call "SeriellRead-11-15.vi"("SkalierungsfaktorHorst"=w545, "VorwortHorst"=w546, "Zwischenspeicher"=w547, "Senden?"=w540, "FPGA VI Reference In"=w528) -> ("Senden?"=w548:bool[], "Zwischenspeicher"=w521:string[])  [unwired: 4 in, 1 out]
          }
        }
      }
      n471 = flat-sequence {
        frame #0 {
          n472 = control-ref of="CO2 B 2"() -> (w335:refnum<vi>)
          n473 = control-ref of="raw data buffer out"() -> (w336:refnum<vi>)
          n474 = control-ref of="manual control"() -> (w337:refnum<vi>)
          n475 = call "licore (main).vi"("manual control"=w337, "raw data"=w336, "Licor-parameter"="command parameter", "graph"=w335) -> ()  [unwired: 8 in]
        }
      }
    }
    frame #2 {
      n476 = xnode "Read/Write Control"("FPGA VI Reference In"=w1203, "global stop"=TRUE) -> ("FPGA VI Reference Out"=w1202:refnum<k20>)  [unwired: 1 in, 1 out]
      n477 = xnode "Close FPGA VI Reference"("FPGA VI Reference In"=w1202) -> ()  [unwired: 1 in, 1 out]
    }
  }
